vi "init Tests.vi"(8 "error in (no error)":errorcluster caption="Fehler (Eingang, kein Fehler)", 11 "EMTestCWS500N Eingang":refnum<class "EMTestCWS500N.lvclass"> caption="DNL_LabVIEW Object in") -> (0 "error out":errorcluster caption="Fehler (Ausgang)", 3 "EMTestCWS500N Ausgang":refnum<class "EMTestCWS500N.lvclass"> caption="DNL_LabVIEW Object out")   [LabVIEW 2013, in "EMTestCWS500N.lvclass"]
uses:
  EMTestCWS500N.lvclass
  Tests/HF-Felder/HF-Felder.lvclass
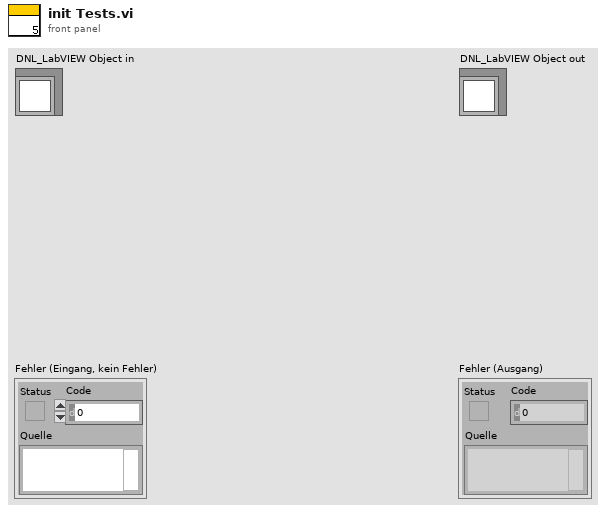
[diagram p1: front panel]
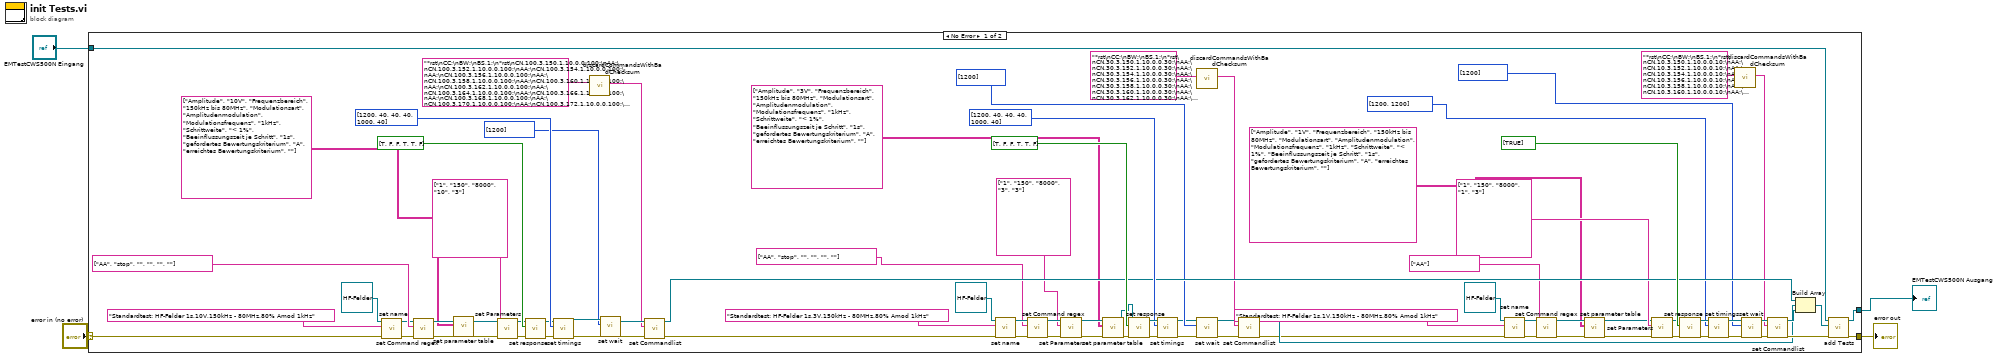
[diagram p0: block diagram]
diagram:
  n1 = case shown="No Error" "error in (no error)" {
    selector: "error in (no error)" -> [w52 w88]
    tunnel: [w76 w88] -> w4
    tunnel: "EMTestCWS500N Eingang" -> [w75 w89]
    tunnel: [w74 w89] -> w1
    frame No Error {
      n2 = call-dynamic "set name.vi"("error in (no error)"=w52, "name"="Standardtest: HF-Felder 1s,10V,150kHz - 80MHz,80% Amod 1kHz", "TestInterface (Eingang)"=refnum<class "HF-Felder.lvclass"> refnum ("HF-Felder.lvclass")) -> ("error out"=w51:errorcluster, "TestInterface (Ausgang)"=w57:refnum<class "HF-Felder.lvclass">)  [unwired: 7 in]
      n3 = call-dynamic "set Command regex.vi"("error in (no error)"=w51, "Command regex"=string[] ["AA", "stop", "", "", "", ""], "TestInterface (Eingang)"=w57) -> ("error out"=w30:errorcluster, "TestInterface (Ausgang)"=w31:refnum<class "HF-Felder.lvclass">)  [unwired: 7 in]
      n4 = call-dynamic "set parameter table.vi"("error in (no error)"=w30, "parameter table"=string[][] [["Amplitude", "10V"], ["Frequenzbereich", "150kHz bis 80MHz"], ["Modulationsart", "Amplitudenmodulation"], ["Modulationsfrequenz", "1kHz"], ["Schrittweite", "< 1%"], ["Beeinflussungszeit je Schritt", "1s"], ["gefordertes Bewertungskriterium", "A"], ["erreichtes Bewertungskriterium", ""]] ("parameters"), "TestInterface in"=w31) -> ("error out"=w29:errorcluster, "TestInterface out"=w28:refnum<class "HF-Felder.lvclass">)  [unwired: 7 in]
      n5 = call-dynamic "set Parameters.vi"("error in (no error)"=w29, "parameters"=string[] ["1", "150", "8000", "10", "3"], "TestInterface (Eingang)"=w28) -> ("error out"=w50:errorcluster, "TestInterface (Ausgang)"=w58:refnum<class "HF-Felder.lvclass">)  [unwired: 7 in]
      n6 = call-dynamic "set response.vi"("error in (no error)"=w50, "response?"=bool[] [TRUE, FALSE, FALSE, TRUE, TRUE, FALSE], "TestInterface (Eingang)"=w58) -> ("error out"=w49:errorcluster, "TestInterface (Ausgang)"=w59:refnum<class "HF-Felder.lvclass">)  [unwired: 7 in]
      n7 = call-dynamic "set timings.vi"("error in (no error)"=w49, "timings"=i32[] [1200, 40, 40, 40, 1000, 40] ("Timings"), "TestInterface (Eingang)"=w59) -> ("error out"=w40:errorcluster, "TestInterface (Ausgang)"=w37:refnum<class "HF-Felder.lvclass">)  [unwired: 7 in]
      n8 = call "discardCommandsWithBadChecksum.vi"("multi-line string"="*rst\nCC;\nBW;\nBS,1;\n*rst\nCN,100,3,150,1,10,0,0,100;\nAA;\nCN,100,3,152,1,10,0,0,100;\nAA;\nCN,100,3,154,1,10,0,0,100;\nAA;\nCN,100,3,156,1,10,0,0,100;\nAA;\nCN,100,3,158,1,10,0,0,100;\nAA;\nCN,100,3,160,1,10,0,0,100;\nAA;\nCN,100,3,162,1,10,0,0,100;\nAA;\nCN,100,3,164,1,10,0,0,100;\nAA;\nCN,100,3,166,1,10,0,0,100;\nAA;\nCN,100,3,168,1,10,0,0,100;\nAA;\nCN,100,3,170,1,10,0,0,100;\nAA;\nCN,100,3,172,1,10,0,0,100;\nAA;\nCN,100,3,174,1,10,0,0,100;\nAA;\nCN,100,3,176,1,10,0,0,100;\nAA;\nCN,100,3,178,1,10,0,0,100;\nAA;\nCN,100,3,180,1,10,0,0,100;\nAA;\nCN,100,3,182,1,10,0,0,100;\nAA;\nCN,100,3,184,1,10,0,0,100;\nAA;\nCN,100,3,186,1,10,0,0,100;\nAA;\nCN,100,3,188,1,10,0,0,100;\nAA;\nCN,100,3,190,1,10,0,0,100;\nAA;\nCN,100,3,192,1,10,0,0,100;\nAA;\nCN,100,3,194,1,10,0,0,100;\nAA;\nCN,100,3,196,1,10,0,0,100;\nAA;\nCN,100,3,198,1,10,0,0,100;\nAA;\nCN,100,3,200,1,10,0,0,100;\nAA;\nCN,100,3,202,1,10,0,0,100;\nAA;\nCN,100,3,204,1,10,0,0,100;\nAA;\nCN,100,3,206,1,10,0,0,100;\nAA;\nCN,100,3,208,1,10,0,0,100;\nAA;\nCN,100,3,210,1,10,0,0,100;\nAA;\nCN,100,3,212,1,10,0,0,100;\nAA;\nCN,100,3,214,1,10,0,0,100;\nAA;\nCN,100,3,216,1,10,0,0,100;\nAA;\nCN,100,3,218,1,10,0,0,100;\nAA;\nCN,100,3,220,1,10,0,0,100;\nAA;\nCN,100,3,222,1,10,0,0,100;\nAA;\nCN,100,3,224,1,10,0,0,100;\nAA;\nCN,100,3,226,1,10,0,0,100;\nAA;\nCN,100,3,228,1,10,0,0,100;\nAA;\nCN,100,3,230,1,10,0,0,100;\nAA;\nCN,100,3,232,1,10,0,0,100;\nAA;\nCN,100,3,234,1,10,0,0,100;\nAA;\nCN,100,3,236,1,10,0,0,100;\nAA;\nCN,100,3,238,1,10,0,0,100;\nAA;\nCN,100,3,240,1,10,0,0,100;\nAA;\nCN,100,3,242,1,10,0,0,100;\nAA;\nCN,100,3,244,1,10,0,0,100;\nAA;\nCN,100,3,246,1,10,0,0,100;\nAA;\nCN,100,3,248,1,10,0,0,100;\nAA;\nCN,100,3,250,1,10,0,0,100;\nAA;\nCN,100,3,252,1,10,0,0,100;\nAA;\nCN,100,3,255,1,10,0,0,100;\nAA;\nCN,100,3,258,1,10,0,0,100;\nAA;\nCN,100,3,261,1,10,0,0,100;\nAA;\nCN,100,3,264,1,10,0,0,100;\nAA;\nCN,100,3,267,1,10,0,0,100;\nAA;\nCN,100,3,270,1,10,0,0,100;\nAA;\nCN,100,3,273,1,10,0,0,100;\nAA;\nCN,100,3,276,1,10,0,0,100;\nAA;\nCN,100,3,279,1,10,0,0,100;\nAA;\nCN,100,3,282,1,10,0,0,100;\nAA;\nCN,100,3,285,1,10,0,0,100;\nAA;\nCN,100,3,288,1,10,0,0,100;\nAA;\nCN,100,3,291,1,10,0,0,100;\nAA;\nCN,100,3,294,1,10,0,0,100;\nAA;\nCN,100,3,297,1,10,0,0,100;\nAA;\nCN,100,3,300,1,10,0,0,100;\nAA;\nCN,100,3,303,1,10,0,0,100;\nAA;\nCN,100,3,306,1,10,0,0,100;\nAA;\nCN,100,3,309,1,10,0,0,100;\nAA;\nCN,100,3,312,1,10,0,0,100;\nAA;\nCN,100,3,315,1,10,0,0,100;\nAA;\nCN,100,3,318,1,10,0,0,100;\nAA;\nCN,100,3,321,1,10,0,0,100;\nAA;\nCN,100,3,324,1,10,0,0,100;\nAA;\nCN,100,3,327,1,10,0,0,100;\nAA;\nCN,100,3,330,1,10,0,0,100;\nAA;\nCN,100,3,333,1,10,0,0,100;\nAA;\nCN,100,3,336,1,10,0,0,100;\nAA;\nCN,100,3,339,1,10,0,0,100;\nAA;\nCN,100,3,342,1,10,0,0,100;\nAA;\nCN,100,3,345,1,10,0,0,100;\nAA;\nCN,100,3,348,1,10,0,0,100;\nAA;\nCN,100,3,351,1,10,0,0,100;\nAA;\nCN,100,3,355,1,10,0,0,100;\nAA;\nCN,100,3,359,1,10,0,0,100;\nAA;\nCN,100,3,363,1,10,0,0,100;\nAA;\nCN,100,3,367,1,10,0,0,100;\nAA;\nCN,100,3,371,1,10,0,0,100;\nAA;\nCN,100,3,375,1,10,0,0,100;\nAA;\nCN,100,3,379,1,10,0,0,100;\nAA;\nCN,100,3,383,1,10,0,0,100;\nAA;\nCN,100,3,387,1,10,0,0,100;\nAA;\nCN,100,3,391,1,10,0,0,100;\nAA;\nCN,100,3,395,1,10,0,0,100;\nAA;\nCN,100,3,399,1,10,0,0,100;\nAA;\nCN,100,3,403,1,10,0,0,100;\nAA;\nCN,100,3,407,1,10,0,0,100;\nAA;\nCN,100,3,411,1,10,0,0,100;\nAA;\nCN,100,3,415,1,10,0,0,100;\nAA;\nCN,100,3,419,1,10,0,0,100;\nAA;\nCN,100,3,423,1,10,0,0,100;\nAA;\nCN,100,3,427,1,10,0,0,100;\nAA;\nCN,100,3,431,1,10,0,0,100;\nAA;\nCN,100,3,435,1,10,0,0,100;\nAA;\nCN,100,3,439,1,10,0,0,100;\nAA;\nCN,100,3,443,1,10,0,0,100;\nAA;\nCN,100,3,447,1,10,0,0,100;\nAA;\nCN,100,3,451,1,10,0,0,100;\nAA;\nCN,100,3,456,1,10,0,0,100;\nAA;\nCN,100,3,461,1,10,0,0,100;\nAA;\nCN,100,3,466,1,10,0,0,100;\nAA;\nCN,100,3,471,1,10,0,0,100;\nAA;\nCN,100,3,476,1,10,0,0,100;\nAA;\nCN,100,3,481,1,10,0,0,100;\nAA;\nCN,100,3,486,1,10,0,0,100;\nAA;\nCN,100,3,491,1,10,0,0,100;\nAA;\nCN,100,3,496,1,10,0,0,100;\nAA;\nCN,100,3,501,1,10,0,0,100;\nAA;\nCN,100,3,506,1,10,0,0,100;\nAA;\nCN,100,3,511,1,10,0,0,100;\nAA;\nCN,100,3,516,1,10,0,0,100;\nAA;\nCN,100,3,521,1,10,0,0,100;\nAA;\nCN,100,3,526,1,10,0,0,100;\nAA;\nCN,100,3,531,1,10,0,0,100;\nAA;\nCN,100,3,536,1,10,0,0,100;\nAA;\nCN,100,3,541,1,10,0,0,100;\nAA;\nCN,100,3,546,1,10,0,0,100;\nAA;\nCN,100,3,551,1,10,0,0,100;\nAA;\nCN,100,3,557,1,10,0,0,100;\nAA;\nCN,100,3,563,1,10,0,0,100;\nAA;\nCN,100,3,569,1,10,0,0,100;\nAA;\nCN,100,3,575,1,10,0,0,100;\nAA;\nCN,100,3,581,1,10,0,0,100;\nAA;\nCN,100,3,587,1,10,0,0,100;\nAA;\nCN,100,3,593,1,10,0,0,100;\nAA;\nCN,100,3,599,1,10,0,0,100;\nAA;\nCN,100,3,605,1,10,0,0,100;\nAA;\nCN,100,3,611,1,10,0,0,100;\nAA;\nCN,100,3,617,1,10,0,0,100;\nAA;\nCN,100,3,623,1,10,0,0,100;\nAA;\nCN,100,3,629,1,10,0,0,100;\nAA;\nCN,100,3,635,1,10,0,0,100;\nAA;\nCN,100,3,641,1,10,0,0,100;\nAA;\nCN,100,3,647,1,10,0,0,100;\nAA;\nCN,100,3,653,1,10,0,0,100;\nAA;\nCN,100,3,660,1,10,0,0,100;\nAA;\nCN,100,3,667,1,10,0,0,100;\nAA;\nCN,100,3,674,1,10,0,0,100;\nAA;\nCN,100,3,681,1,10,0,0,100;\nAA;\nCN,100,3,688,1,10,0,0,100;\nAA;\nCN,100,3,695,1,10,0,0,100;\nAA;\nCN,100,3,702,1,10,0,0,100;\nAA;\nCN,100,3,709,1,10,0,0,100;\nAA;\nCN,100,3,716,1,10,0,0,100;\nAA;\nCN,100,3,723,1,10,0,0,100;\nAA;\nCN,100,3,730,1,10,0,0,100;\nAA;\nCN,100,3,737,1,10,0,0,100;\nAA;\nCN,100,3,744,1,10,0,0,100;\nAA;\nCN,100,3,751,1,10,0,0,100;\nAA;\nCN,100,3,759,1,10,0,0,100;\nAA;\nCN,100,3,767,1,10,0,0,100;\nAA;\nCN,100,3,775,1,10,0,0,100;\nAA;\nCN,100,3,783,1,10,0,0,100;\nAA;\nCN,100,3,791,1,10,0,0,100;\nAA;\nCN,100,3,799,1,10,0,0,100;\nAA;\nCN,100,3,807,1,10,0,0,100;\nAA;\nCN,100,3,815,1,10,0,0,100;\nAA;\nCN,100,3,823,1,10,0,0,100;\nAA;\nCN,100,3,831,1,10,0,0,100;\nAA;\nCN,100,3,839,1,10,0,0,100;\nAA;\nCN,100,3,847,1,10,0,0,100;\nAA;\nCN,100,3,855,1,10,0,0,100;\nAA;\nCN,100,3,864,1,10,0,0,100;\nAA;\nCN,100,3,873,1,10,0,0,100;\nAA;\nCN,100,3,882,1,10,0,0,100;\nAA;\nCN,100,3,891,1,10,0,0,100;\nAA;\nCN,100,3,900,1,10,0,0,100;\nAA;\nCN,100,3,909,1,10,0,0,100;\nAA;\nCN,100,3,918,1,10,0,0,100;\nAA;\nCN,100,3,927,1,10,0,0,100;\nAA;\nCN,100,3,936,1,10,0,0,100;\nAA;\nCN,100,3,945,1,10,0,0,100;\nAA;\nCN,100,3,954,1,10,0,0,100;\nAA;\nCN,100,3,964,1,10,0,0,100;\nAA;\nCN,100,3,974,1,10,0,0,100;\nAA;\nCN,100,3,984,1,10,0,0,100;\nAA;\nCN,100,3,994,1,10,0,0,100;\nAA;\nCN,100,3,1004,1,10,0,0,100;\nAA;\nCN,100,3,1014,1,10,0,0,100;\nAA;\nCN,100,3,1024,1,10,0,0,100;\nAA;\nCN,100,3,1034,1,10,0,0,100;\nAA;\nCN,100,3,1044,1,10,0,0,100;\nAA;\nCN,100,3,1054,1,10,0,0,100;\nAA;\nCN,100,3,1065,1,10,0,0,100;\nAA;\nCN,100,3,1076,1,10,0,0,100;\nAA;\nCN,100,3,1087,1,10,0,0,100;\nAA;\nCN,100,3,1098,1,10,0,0,100;\nAA;\nCN,100,3,1109,1,10,0,0,100;\nAA;\nCN,100,3,1120,1,10,0,0,100;\nAA;\nCN,100,3,1131,1,10,0,0,100;\nAA;\nCN,100,3,1142,1,10,0,0,100;\nAA;\nCN,100,3,1153,1,10,0,0,100;\nAA;\nCN,100,3,1165,1,10,0,0,100;\nAA;\nCN,100,3,1177,1,10,0,0,100;\nAA;\nCN,100,3,1189,1,10,0,0,100;\nAA;\nCN,100,3,1201,1,10,0,0,100;\nAA;\nCN,100,3,1213,1,10,0,0,100;\nAA;\nCN,100,3,1225,1,10,0,0,100;\nAA;\nCN,100,3,1237,1,10,0,0,100;\nAA;\nCN,100,3,1249,1,10,0,0,100;\nAA;\nCN,100,3,1261,1,10,0,0,100;\nAA;\nCN,100,3,1274,1,10,0,0,100;\nAA;\nCN,100,3,1287,1,10,0,0,100;\nAA;\nCN,100,3,1300,1,10,0,0,100;\nAA;\nCN,100,3,1313,1,10,0,0,100;\nAA;\nCN,100,3,1326,1,10,0,0,100;\nAA;\nCN,100,3,1339,1,10,0,0,100;\nAA;\nCN,100,3,1352,1,10,0,0,100;\nAA;\nCN,100,3,1366,1,10,0,0,100;\nAA;\nCN,100,3,1380,1,10,0,0,100;\nAA;\nCN,100,3,1394,1,10,0,0,100;\nAA;\nCN,100,3,1408,1,10,0,0,100;\nAA;\nCN,100,3,1422,1,10,0,0,100;\nAA;\nCN,100,3,1436,1,10,0,0,100;\nAA;\nCN,100,3,1450,1,10,0,0,100;\nAA;\nCN,100,3,1464,1,10,0,0,100;\nAA;\nCN,100,3,1479,1,10,0,0,100;\nAA;\nCN,100,3,1494,1,10,0,0,100;\nAA;\nCN,100,3,1509,1,10,0,0,100;\nAA;\nCN,100,3,1524,1,10,0,0,100;\nAA;\nCN,100,3,1539,1,10,0,0,100;\nAA;\nCN,100,3,1554,1,10,0,0,100;\nAA;\nCN,100,3,1570,1,10,0,0,100;\nAA;\nCN,100,3,1586,1,10,0,0,100;\nAA;\nCN,100,3,1602,1,10,0,0,100;\nAA;\nCN,100,3,1618,1,10,0,0,100;\nAA;\nCN,100,3,1634,1,10,0,0,100;\nAA;\nCN,100,3,1650,1,10,0,0,100;\nAA;\nCN,100,3,1666,1,10,0,0,100;\nAA;\nCN,100,3,1683,1,10,0,0,100;\nAA;\nCN,100,3,1700,1,10,0,0,100;\nAA;\nCN,100,3,1717,1,10,0,0,100;\nAA;\nCN,100,3,1734,1,10,0,0,100;\nAA;\nCN,100,3,1751,1,10,0,0,100;\nAA;\nCN,100,3,1769,1,10,0,0,100;\nAA;\nCN,100,3,1787,1,10,0,0,100;\nAA;\nCN,100,3,1805,1,10,0,0,100;\nAA;\nCN,100,3,1823,1,10,0,0,100;\nAA;\nCN,100,3,1841,1,10,0,0,100;\nAA;\nCN,100,3,1859,1,10,0,0,100;\nAA;\nCN,100,3,1878,1,10,0,0,100;\nAA;\nCN,100,3,1897,1,10,0,0,100;\nAA;\nCN,100,3,1916,1,10,0,0,100;\nAA;\nCN,100,3,1935,1,10,0,0,100;\nAA;\nCN,100,3,1954,1,10,0,0,100;\nAA;\nCN,100,3,1974,1,10,0,0,100;\nAA;\nCN,100,3,1994,1,10,0,0,100;\nAA;\nCN,100,3,2014,1,10,0,0,100;\nAA;\nCN,100,3,2034,1,10,0,0,100;\nAA;\nCN,100,3,2054,1,10,0,0,100;\nAA;\nCN,100,3,2075,1,10,0,0,100;\nAA;\nCN,100,3,2096,1,10,0,0,100;\nAA;\nCN,100,3,2117,1,10,0,0,100;\nAA;\nCN,100,3,2138,1,10,0,0,100;\nAA;\nCN,100,3,2159,1,10,0,0,100;\nAA;\nCN,100,3,2181,1,10,0,0,100;\nAA;\nCN,100,3,2203,1,10,0,0,100;\nAA;\nCN,100,3,2225,1,10,0,0,100;\nAA;\nCN,100,3,2247,1,10,0,0,100;\nAA;\nCN,100,3,2269,1,10,0,0,100;\nAA;\nCN,100,3,2292,1,10,0,0,100;\nAA;\nCN,100,3,2315,1,10,0,0,100;\nAA;\nCN,100,3,2338,1,10,0,0,100;\nAA;\nCN,100,3,2361,1,10,0,0,100;\nAA;\nCN,100,3,2385,1,10,0,0,100;\nAA;\nCN,100,3,2409,1,10,0,0,100;\nAA;\nCN,100,3,2433,1,10,0,0,100;\nAA;\nCN,100,3,2457,1,10,0,0,100;\nAA;\nCN,100,3,2482,1,10,0,0,100;\nAA;\nCN,100,3,2507,1,10,0,0,100;\nAA;\nCN,100,3,2532,1,10,0,0,100;\nAA;\nCN,100,3,2557,1,10,0,0,100;\nAA;\nCN,100,3,2583,1,10,0,0,100;\nAA;\nCN,100,3,2609,1,10,0,0,100;\nAA;\nCN,100,3,2635,1,10,0,0,100;\nAA;\nCN,100,3,2661,1,10,0,0,100;\nAA;\nCN,100,3,2688,1,10,0,0,100;\nAA;\nCN,100,3,2715,1,10,0,0,100;\nAA;\nCN,100,3,2742,1,10,0,0,100;\nAA;\nCN,100,3,2769,1,10,0,0,100;\nAA;\nCN,100,3,2797,1,10,0,0,100;\nAA;\nCN,100,3,2825,1,10,0,0,100;\nAA;\nCN,100,3,2853,1,10,0,0,100;\nAA;\nCN,100,3,2882,1,10,0,0,100;\nAA;\nCN,100,3,2911,1,10,0,0,100;\nAA;\nCN,100,3,2940,1,10,0,0,100;\nAA;\nCN,100,3,2969,1,10,0,0,100;\nAA;\nCN,100,3,2999,1,10,0,0,100;\nAA;\nCN,100,3,3029,1,10,0,0,100;\nAA;\nCN,100,3,3059,1,10,0,0,100;\nAA;\nCN,100,3,3090,1,10,0,0,100;\nAA;\nCN,100,3,3121,1,10,0,0,100;\nAA;\nCN,100,3,3152,1,10,0,0,100;\nAA;\nCN,100,3,3184,1,10,0,0,100;\nAA;\nCN,100,3,3216,1,10,0,0,100;\nAA;\nCN,100,3,3248,1,10,0,0,100;\nAA;\nCN,100,3,3280,1,10,0,0,100;\nAA;\nCN,100,3,3313,1,10,0,0,100;\nAA;\nCN,100,3,3346,1,10,0,0,100;\nAA;\nCN,100,3,3379,1,10,0,0,100;\nAA;\nCN,100,3,3413,1,10,0,0,100;\nAA;\nCN,100,3,3447,1,10,0,0,100;\nAA;\nCN,100,3,3481,1,10,0,0,100;\nAA;\nCN,100,3,3516,1,10,0,0,100;\nAA;\nCN,100,3,3551,1,10,0,0,100;\nAA;\nCN,100,3,3587,1,10,0,0,100;\nAA;\nCN,100,3,3623,1,10,0,0,100;\nAA;\nCN,100,3,3659,1,10,0,0,100;\nAA;\nCN,100,3,3696,1,10,0,0,100;\nAA;\nCN,100,3,3733,1,10,0,0,100;\nAA;\nCN,100,3,3770,1,10,0,0,100;\nAA;\nCN,100,3,3808,1,10,0,0,100;\nAA;\nCN,100,3,3846,1,10,0,0,100;\nAA;\nCN,100,3,3884,1,10,0,0,100;\nAA;\nCN,100,3,3923,1,10,0,0,100;\nAA;\nCN,100,3,3962,1,10,0,0,100;\nAA;\nCN,100,3,4002,1,10,0,0,100;\nAA;\nCN,100,3,4042,1,10,0,0,100;\nAA;\nCN,100,3,4082,1,10,0,0,100;\nAA;\nCN,100,3,4123,1,10,0,0,100;\nAA;\nCN,100,3,4164,1,10,0,0,100;\nAA;\nCN,100,3,4206,1,10,0,0,100;\nAA;\nCN,100,3,4248,1,10,0,0,100;\nAA;\nCN,100,3,4290,1,10,0,0,100;\nAA;\nCN,100,3,4333,1,10,0,0,100;\nAA;\nCN,100,3,4376,1,10,0,0,100;\nAA;\nCN,100,3,4420,1,10,0,0,100;\nAA;\nCN,100,3,4464,1,10,0,0,100;\nAA;\nCN,100,3,4509,1,10,0,0,100;\nAA;\nCN,100,3,4554,1,10,0,0,100;\nAA;\nCN,100,3,4600,1,10,0,0,100;\nAA;\nCN,100,3,4646,1,10,0,0,100;\nAA;\nCN,100,3,4692,1,10,0,0,100;\nAA;\nCN,100,3,4739,1,10,0,0,100;\nAA;\nCN,100,3,4786,1,10,0,0,100;\nAA;\nCN,100,3,4834,1,10,0,0,100;\nAA;\nCN,100,3,4882,1,10,0,0,100;\nAA;\nCN,100,3,4931,1,10,0,0,100;\nAA;\nCN,100,3,4980,1,10,0,0,100;\nAA;\nCN,100,3,5030,1,10,0,0,100;\nAA;\nCN,100,3,5080,1,10,0,0,100;\nAA;\nCN,100,3,5131,1,10,0,0,100;\nAA;\nCN,100,3,5182,1,10,0,0,100;\nAA;\nCN,100,3,5234,1,10,0,0,100;\nAA;\nCN,100,3,5286,1,10,0,0,100;\nAA;\nCN,100,3,5339,1,10,0,0,100;\nAA;\nCN,100,3,5392,1,10,0,0,100;\nAA;\nCN,100,3,5446,1,10,0,0,100;\nAA;\nCN,100,3,5500,1,10,0,0,100;\nAA;\nCN,100,3,5555,1,10,0,0,100;\nAA;\nCN,100,3,5611,1,10,0,0,100;\nAA;\nCN,100,3,5667,1,10,0,0,100;\nAA;\nCN,100,3,5724,1,10,0,0,100;\nAA;\nCN,100,3,5781,1,10,0,0,100;\nAA;\nCN,100,3,5839,1,10,0,0,100;\nAA;\nCN,100,3,5897,1,10,0,0,100;\nAA;\nCN,100,3,5956,1,10,0,0,100;\nAA;\nCN,100,3,6016,1,10,0,0,100;\nAA;\nCN,100,3,6076,1,10,0,0,100;\nAA;\nCN,100,3,6137,1,10,0,0,100;\nAA;\nCN,100,3,6198,1,10,0,0,100;\nAA;\nCN,100,3,6260,1,10,0,0,100;\nAA;\nCN,100,3,6323,1,10,0,0,100;\nAA;\nCN,100,3,6386,1,10,0,0,100;\nAA;\nCN,100,3,6450,1,10,0,0,100;\nAA;\nCN,100,3,6514,1,10,0,0,100;\nAA;\nCN,100,3,6579,1,10,0,0,100;\nAA;\nCN,100,3,6645,1,10,0,0,100;\nAA;\nCN,100,3,6711,1,10,0,0,100;\nAA;\nCN,100,3,6778,1,10,0,0,100;\nAA;\nCN,100,3,6846,1,10,0,0,100;\nAA;\nCN,100,3,6914,1,10,0,0,100;\nAA;\nCN,100,3,6983,1,10,0,0,100;\nAA;\nCN,100,3,7053,1,10,0,0,100;\nAA;\nCN,100,3,7124,1,10,0,0,100;\nAA;\nCN,100,3,7195,1,10,0,0,100;\nAA;\nCN,100,3,7267,1,10,0,0,100;\nAA;\nCN,100,3,7340,1,10,0,0,100;\nAA;\nCN,100,3,7413,1,10,0,0,100;\nAA;\nCN,100,3,7487,1,10,0,0,100;\nAA;\nCN,100,3,7562,1,10,0,0,100;\nAA;\nCN,100,3,7638,1,10,0,0,100;\nAA;\nCN,100,3,7714,1,10,0,0,100;\nAA;\nCN,100,3,7791,1,10,0,0,100;\nAA;\nCN,100,3,7869,1,10,0,0,100;\nAA;\nCN,100,3,7948,1,10,0,0,100;\nAA;\nCN,100,3,8027,1,10,0,0,100;\nAA;\nCN,100,3,8107,1,10,0,0,100;\nAA;\nCN,100,3,8188,1,10,0,0,100;\nAA;\nCN,100,3,8270,1,10,0,0,100;\nAA;\nCN,100,3,8353,1,10,0,0,100;\nAA;\nCN,100,3,8437,1,10,0,0,100;\nAA;\nCN,100,3,8521,1,10,0,0,100;\nAA;\nCN,100,3,8606,1,10,0,0,100;\nAA;\nCN,100,3,8692,1,10,0,0,100;\nAA;\nCN,100,3,8779,1,10,0,0,100;\nAA;\nCN,100,3,8867,1,10,0,0,100;\nAA;\nCN,100,3,8956,1,10,0,0,100;\nAA;\nCN,100,3,9046,1,10,0,0,100;\nAA;\nCN,100,3,9136,1,10,0,0,100;\nAA;\nCN,100,3,9227,1,10,0,0,100;\nAA;\nCN,100,3,9319,1,10,0,0,100;\nAA;\nCN,100,3,9412,1,10,0,0,100;\nAA;\nCN,100,3,9506,1,10,0,0,100;\nAA;\nCN,100,3,9601,1,10,0,0,100;\nAA;\nCN,100,3,9697,1,10,0,0,100;\nAA;\nCN,100,3,9794,1,10,0,0,100;\nAA;\nCN,100,3,9892,1,10,0,0,100;\nAA;\nCN,100,3,9991,1,10,0,0,100;\nAA;\nCN,100,3,10091,1,10,0,0,100;\nAA;\nCN,100,3,10192,1,10,0,0,100;\nAA;\nCN,100,3,10294,1,10,0,0,100;\nAA;\nCN,100,3,10397,1,10,0,0,100;\nAA;\nCN,100,3,10501,1,10,0,0,100;\nAA;\nCN,100,3,10606,1,10,0,0,100;\nAA;\nCN,100,3,10712,1,10,0,0,100;\nAA;\nCN,100,3,10819,1,10,0,0,100;\nAA;\nCN,100,3,10927,1,10,0,0,100;\nAA;\nCN,100,3,11036,1,10,0,0,100;\nAA;\nCN,100,3,11146,1,10,0,0,100;\nAA;\nCN,100,3,11257,1,10,0,0,100;\nAA;\nCN,100,3,11370,1,10,0,0,100;\nAA;\nCN,100,3,11484,1,10,0,0,100;\nAA;\nCN,100,3,11599,1,10,0,0,100;\nAA;\nCN,100,3,11715,1,10,0,0,100;\nAA;\nCN,100,3,11832,1,10,0,0,100;\nAA;\nCN,100,3,11950,1,10,0,0,100;\nAA;\nCN,100,3,12070,1,10,0,0,100;\nAA;\nCN,100,3,12191,1,10,0,0,100;\nAA;\nCN,100,3,12313,1,10,0,0,100;\nAA;\nCN,100,3,12436,1,10,0,0,100;\nAA;\nCN,100,3,12560,1,10,0,0,100;\nAA;\nCN,100,3,12686,1,10,0,0,100;\nAA;\nCN,100,3,12813,1,10,0,0,100;\nAA;\nCN,100,3,12941,1,10,0,0,100;\nAA;\nCN,100,3,13070,1,10,0,0,100;\nAA;\nCN,100,3,13201,1,10,0,0,100;\nAA;\nCN,100,3,13333,1,10,0,0,100;\nAA;\nCN,100,3,13466,1,10,0,0,100;\nAA;\nCN,100,3,13601,1,10,0,0,100;\nAA;\nCN,100,3,13737,1,10,0,0,100;\nAA;\nCN,100,3,13874,1,10,0,0,100;\nAA;\nCN,100,3,14013,1,10,0,0,100;\nAA;\nCN,100,3,14153,1,10,0,0,100;\nAA;\nCN,100,3,14295,1,10,0,0,100;\nAA;\nCN,100,3,14438,1,10,0,0,100;\nAA;\nCN,100,3,14582,1,10,0,0,100;\nAA;\nCN,100,3,14728,1,10,0,0,100;\nAA;\nCN,100,3,14875,1,10,0,0,100;\nAA;\nCN,100,3,15024,1,10,0,0,100;\nAA;\nCN,100,3,15174,1,10,0,0,100;\nAA;\nCN,100,3,15326,1,10,0,0,100;\nAA;\nCN,100,3,15479,1,10,0,0,100;\nAA;\nCN,100,3,15634,1,10,0,0,100;\nAA;\nCN,100,3,15790,1,10,0,0,100;\nAA;\nCN,100,3,15948,1,10,0,0,100;\nAA;\nCN,100,3,16107,1,10,0,0,100;\nAA;\nCN,100,3,16268,1,10,0,0,100;\nAA;\nCN,100,3,16431,1,10,0,0,100;\nAA;\nCN,100,3,16595,1,10,0,0,100;\nAA;\nCN,100,3,16761,1,10,0,0,100;\nAA;\nCN,100,3,16929,1,10,0,0,100;\nAA;\nCN,100,3,17098,1,10,0,0,100;\nAA;\nCN,100,3,17269,1,10,0,0,100;\nAA;\nCN,100,3,17442,1,10,0,0,100;\nAA;\nCN,100,3,17616,1,10,0,0,100;\nAA;\nCN,100,3,17792,1,10,0,0,100;\nAA;\nCN,100,3,17970,1,10,0,0,100;\nAA;\nCN,100,3,18150,1,10,0,0,100;\nAA;\nCN,100,3,18332,1,10,0,0,100;\nAA;\nCN,100,3,18515,1,10,0,0,100;\nAA;\nCN,100,3,18700,1,10,0,0,100;\nAA;\nCN,100,3,18887,1,10,0,0,100;\nAA;\nCN,100,3,19076,1,10,0,0,100;\nAA;\nCN,100,3,19267,1,10,0,0,100;\nAA;\nCN,100,3,19460,1,10,0,0,100;\nAA;\nCN,100,3,19655,1,10,0,0,100;\nAA;\nCN,100,3,19852,1,10,0,0,100;\nAA;\nCN,100,3,20051,1,10,0,0,100;\nAA;\nCN,100,3,20252,1,10,0,0,100;\nAA;\nCN,100,3,20455,1,10,0,0,100;\nAA;\nCN,100,3,20660,1,10,0,0,100;\nAA;\nCN,100,3,20867,1,10,0,0,100;\nAA;\nCN,100,3,21076,1,10,0,0,100;\nAA;\nCN,100,3,21287,1,10,0,0,100;\nAA;\nCN,100,3,21500,1,10,0,0,100;\nAA;\nCN,100,3,21715,1,10,0,0,100;\nAA;\nCN,100,3,21932,1,10,0,0,100;\nAA;\nCN,100,3,22151,1,10,0,0,100;\nAA;\nCN,100,3,22373,1,10,0,0,100;\nAA;\nCN,100,3,22597,1,10,0,0,100;\nAA;\nCN,100,3,22823,1,10,0,0,100;\nAA;\nCN,100,3,23051,1,10,0,0,100;\nAA;\nCN,100,3,23282,1,10,0,0,100;\nAA;\nCN,100,3,23515,1,10,0,0,100;\nAA;\nCN,100,3,23750,1,10,0,0,100;\nAA;\nCN,100,3,23988,1,10,0,0,100;\nAA;\nCN,100,3,24228,1,10,0,0,100;\nAA;\nCN,100,3,24470,1,10,0,0,100;\nAA;\nCN,100,3,24715,1,10,0,0,100;\nAA;\nCN,100,3,24962,1,10,0,0,100;\nAA;\nCN,100,3,25212,1,10,0,0,100;\nAA;\nCN,100,3,25464,1,10,0,0,100;\nAA;\nCN,100,3,25719,1,10,0,0,100;\nAA;\nCN,100,3,25976,1,10,0,0,100;\nAA;\nCN,100,3,26236,1,10,0,0,100;\nAA;\nCN,100,3,26498,1,10,0,0,100;\nAA;\nCN,100,3,26763,1,10,0,0,100;\nAA;\nCN,100,3,27031,1,10,0,0,100;\nAA;\nCN,100,3,27301,1,10,0,0,100;\nAA;\nCN,100,3,27574,1,10,0,0,100;\nAA;\nCN,100,3,27850,1,10,0,0,100;\nAA;\nCN,100,3,28128,1,10,0,0,100;\nAA;\nCN,100,3,28409,1,10,0,0,100;\nAA;\nCN,100,3,28693,1,10,0,0,100;\nAA;\nCN,100,3,28980,1,10,0,0,100;\nAA;\nCN,100,3,29270,1,10,0,0,100;\nAA;\nCN,100,3,29563,1,10,0,0,100;\nAA;\nCN,100,3,29859,1,10,0,0,100;\nAA;\nCN,100,3,30158,1,10,0,0,100;\nAA;\nCN,100,3,30460,1,10,0,0,100;\nAA;\nCN,100,3,30765,1,10,0,0,100;\nAA;\nCN,100,3,31073,1,10,0,0,100;\nAA;\nCN,100,3,31384,1,10,0,0,100;\nAA;\nCN,100,3,31698,1,10,0,0,100;\nAA;\nCN,100,3,32015,1,10,0,0,100;\nAA;\nCN,100,3,32335,1,10,0,0,100;\nAA;\nCN,100,3,32658,1,10,0,0,100;\nAA;\nCN,100,3,32985,1,10,0,0,100;\nAA;\nCN,100,3,33315,1,10,0,0,100;\nAA;\nCN,100,3,33648,1,10,0,0,100;\nAA;\nCN,100,3,33984,1,10,0,0,100;\nAA;\nCN,100,3,34324,1,10,0,0,100;\nAA;\nCN,100,3,34667,1,10,0,0,100;\nAA;\nCN,100,3,35014,1,10,0,0,100;\nAA;\nCN,100,3,35364,1,10,0,0,100;\nAA;\nCN,100,3,35718,1,10,0,0,100;\nAA;\nCN,100,3,36075,1,10,0,0,100;\nAA;\nCN,100,3,36436,1,10,0,0,100;\nAA;\nCN,100,3,36800,1,10,0,0,100;\nAA;\nCN,100,3,37168,1,10,0,0,100;\nAA;\nCN,100,3,37540,1,10,0,0,100;\nAA;\nCN,100,3,37915,1,10,0,0,100;\nAA;\nCN,100,3,38294,1,10,0,0,100;\nAA;\nCN,100,3,38677,1,10,0,0,100;\nAA;\nCN,100,3,39064,1,10,0,0,100;\nAA;\nCN,100,3,39455,1,10,0,0,100;\nAA;\nCN,100,3,39850,1,10,0,0,100;\nAA;\nCN,100,3,40248,1,10,0,0,100;\nAA;\nCN,100,3,40650,1,10,0,0,100;\nAA;\nCN,100,3,41056,1,10,0,0,100;\nAA;\nCN,100,3,41467,1,10,0,0,100;\nAA;\nCN,100,3,41882,1,10,0,0,100;\nAA;\nCN,100,3,42301,1,10,0,0,100;\nAA;\nCN,100,3,42724,1,10,0,0,100;\nAA;\nCN,100,3,43151,1,10,0,0,100;\nAA;\nCN,100,3,43583,1,10,0,0,100;\nAA;\nCN,100,3,44019,1,10,0,0,100;\nAA;\nCN,100,3,44459,1,10,0,0,100;\nAA;\nCN,100,3,44904,1,10,0,0,100;\nAA;\nCN,100,3,45353,1,10,0,0,100;\nAA;\nCN,100,3,45807,1,10,0,0,100;\nAA;\nCN,100,3,46265,1,10,0,0,100;\nAA;\nCN,100,3,46728,1,10,0,0,100;\nAA;\nCN,100,3,47195,1,10,0,0,100;\nAA;\nCN,100,3,47667,1,10,0,0,100;\nAA;\nCN,100,3,48144,1,10,0,0,100;\nAA;\nCN,100,3,48625,1,10,0,0,100;\nAA;\nCN,100,3,49111,1,10,0,0,100;\nAA;\nCN,100,3,49602,1,10,0,0,100;\nAA;\nCN,100,3,50098,1,10,0,0,100;\nAA;\nCN,100,3,50599,1,10,0,0,100;\nAA;\nCN,100,3,51105,1,10,0,0,100;\nAA;\nCN,100,3,51616,1,10,0,0,100;\nAA;\nCN,100,3,52132,1,10,0,0,100;\nAA;\nCN,100,3,52653,1,10,0,0,100;\nAA;\nCN,100,3,53180,1,10,0,0,100;\nAA;\nCN,100,3,53712,1,10,0,0,100;\nAA;\nCN,100,3,54249,1,10,0,0,100;\nAA;\nCN,100,3,54791,1,10,0,0,100;\nAA;\nCN,100,3,55339,1,10,0,0,100;\nAA;\nCN,100,3,55892,1,10,0,0,100;\nAA;\nCN,100,3,56451,1,10,0,0,100;\nAA;\nCN,100,3,57016,1,10,0,0,100;\nAA;\nCN,100,3,57586,1,10,0,0,100;\nAA;\nCN,100,3,58162,1,10,0,0,100;\nAA;\nCN,100,3,58744,1,10,0,0,100;\nAA;\nCN,100,3,59331,1,10,0,0,100;\nAA;\nCN,100,3,59924,1,10,0,0,100;\nAA;\nCN,100,3,60523,1,10,0,0,100;\nAA;\nCN,100,3,61128,1,10,0,0,100;\nAA;\nCN,100,3,61739,1,10,0,0,100;\nAA;\nCN,100,3,62356,1,10,0,0,100;\nAA;\nCN,100,3,62980,1,10,0,0,100;\nAA;\nCN,100,3,63610,1,10,0,0,100;\nAA;\nCN,100,3,64246,1,10,0,0,100;\nAA;\nCN,100,3,64888,1,10,0,0,100;\nAA;\nCN,100,3,65537,1,10,0,0,100;\nAA;\nCN,100,3,66192,1,10,0,0,100;\nAA;\nCN,100,3,66854,1,10,0,0,100;\nAA;\nCN,100,3,67523,1,10,0,0,100;\nAA;\nCN,100,3,68198,1,10,0,0,100;\nAA;\nCN,100,3,68880,1,10,0,0,100;\nAA;\nCN,100,3,69569,1,10,0,0,100;\nAA;\nCN,100,3,70265,1,10,0,0,100;\nAA;\nCN,100,3,70968,1,10,0,0,100;\nAA;\nCN,100,3,71678,1,10,0,0,100;\nAA;\nCN,100,3,72395,1,10,0,0,100;\nAA;\nCN,100,3,73119,1,10,0,0,100;\nAA;\nCN,100,3,73850,1,10,0,0,100;\nAA;\nCN,100,3,74588,1,10,0,0,100;\nAA;\nCN,100,3,75334,1,10,0,0,100;\nAA;\nCN,100,3,76087,1,10,0,0,100;\nAA;\nCN,100,3,76848,1,10,0,0,100;\nAA;\nCN,100,3,77616,1,10,0,0,100;\nAA;\nCN,100,3,78392,1,10,0,0,100;\nAA;\nCN,100,3,79176,1,10,0,0,100;\nAA;\nCN,100,3,79968,1,10,0,0,100;\nAA;\nCN,100,3,80000,1,10,0,0,100;\nAA;\nAR;" ("Commandlist")) -> ("outputstring"=w10:string)  [unwired: 10 in]
      n9 = call-dynamic "set wait.vi"("error in (no error)"=w40, "wait"=i32[] [1200], "TestInterface in"=w37) -> ("error out"=w39:errorcluster, "TestInterface out"=w38:refnum<class "HF-Felder.lvclass">)  [unwired: 7 in]
      n10 = call-dynamic "set Commandlist.vi"("error in (no error)"=w39, "Commandlist"=w10, "TestInterface (Eingang)"=w38) -> ("error out"=w48:errorcluster, "TestInterface (Ausgang)"=w55:refnum<class "HF-Felder.lvclass">)  [unwired: 7 in]
      n11 = call-dynamic "set name.vi"("error in (no error)"=w48, "name"="Standardtest: HF-Felder 1s,3V,150kHz - 80MHz,80% Amod 1kHz", "TestInterface (Eingang)"=refnum<class "HF-Felder.lvclass"> refnum ("HF-Felder.lvclass")) -> ("error out"=w69:errorcluster, "TestInterface (Ausgang)"=w71:refnum<class "HF-Felder.lvclass">)  [unwired: 7 in]
      n12 = call-dynamic "set Command regex.vi"("error in (no error)"=w69, "Command regex"=string[] ["AA", "stop", "", "", "", ""], "TestInterface (Eingang)"=w71) -> ("error out"=w25:errorcluster, "TestInterface (Ausgang)"=w24:refnum<class "HF-Felder.lvclass">)  [unwired: 7 in]
      n13 = call-dynamic "set Parameters.vi"("error in (no error)"=w25, "parameters"=string[] ["1", "150", "8000", "3", "3"], "TestInterface (Eingang)"=w24) -> ("error out"=w18:errorcluster, "TestInterface (Ausgang)"=w20:refnum<class "HF-Felder.lvclass">)  [unwired: 7 in]
      n14 = call-dynamic "set parameter table.vi"("error in (no error)"=w18, "parameter table"=string[][] [["Amplitude", "3V"], ["Frequenzbereich", "150kHz bis 80MHz"], ["Modulationsart", "Amplitudenmodulation"], ["Modulationsfrequenz", "1kHz"], ["Schrittweite", "< 1%"], ["Beeinflussungszeit je Schritt", "1s"], ["gefordertes Bewertungskriterium", "A"], ["erreichtes Bewertungskriterium", ""]] ("parameters"), "TestInterface in"=w20) -> ("error out"=w22:errorcluster, "TestInterface out"=w21:refnum<class "HF-Felder.lvclass">)  [unwired: 7 in]
      n15 = call-dynamic "set response.vi"("error in (no error)"=w22, "response?"=bool[] [TRUE, FALSE, FALSE, TRUE, TRUE, FALSE], "TestInterface (Eingang)"=w21) -> ("error out"=w68:errorcluster, "TestInterface (Ausgang)"=w70:refnum<class "HF-Felder.lvclass">)  [unwired: 7 in]
      n16 = call-dynamic "set timings.vi"("error in (no error)"=w68, "timings"=i32[] [1200, 40, 40, 40, 1000, 40] ("Timings"), "TestInterface (Eingang)"=w70) -> ("error out"=w33:errorcluster, "TestInterface (Ausgang)"=w34:refnum<class "HF-Felder.lvclass">)  [unwired: 7 in]
      n17 = call "discardCommandsWithBadChecksum.vi"("multi-line string"="*rst\nCC;\nBW;\nBS,1;\n*rst\nCN,30,3,150,1,10,0,0,30;\nAA;\nCN,30,3,152,1,10,0,0,30;\nAA;\nCN,30,3,154,1,10,0,0,30;\nAA;\nCN,30,3,156,1,10,0,0,30;\nAA;\nCN,30,3,158,1,10,0,0,30;\nAA;\nCN,30,3,160,1,10,0,0,30;\nAA;\nCN,30,3,162,1,10,0,0,30;\nAA;\nCN,30,3,164,1,10,0,0,30;\nAA;\nCN,30,3,166,1,10,0,0,30;\nAA;\nCN,30,3,168,1,10,0,0,30;\nAA;\nCN,30,3,170,1,10,0,0,30;\nAA;\nCN,30,3,172,1,10,0,0,30;\nAA;\nCN,30,3,174,1,10,0,0,30;\nAA;\nCN,30,3,176,1,10,0,0,30;\nAA;\nCN,30,3,178,1,10,0,0,30;\nAA;\nCN,30,3,180,1,10,0,0,30;\nAA;\nCN,30,3,182,1,10,0,0,30;\nAA;\nCN,30,3,184,1,10,0,0,30;\nAA;\nCN,30,3,186,1,10,0,0,30;\nAA;\nCN,30,3,188,1,10,0,0,30;\nAA;\nCN,30,3,190,1,10,0,0,30;\nAA;\nCN,30,3,192,1,10,0,0,30;\nAA;\nCN,30,3,194,1,10,0,0,30;\nAA;\nCN,30,3,196,1,10,0,0,30;\nAA;\nCN,30,3,198,1,10,0,0,30;\nAA;\nCN,30,3,200,1,10,0,0,30;\nAA;\nCN,30,3,202,1,10,0,0,30;\nAA;\nCN,30,3,204,1,10,0,0,30;\nAA;\nCN,30,3,206,1,10,0,0,30;\nAA;\nCN,30,3,208,1,10,0,0,30;\nAA;\nCN,30,3,210,1,10,0,0,30;\nAA;\nCN,30,3,212,1,10,0,0,30;\nAA;\nCN,30,3,214,1,10,0,0,30;\nAA;\nCN,30,3,216,1,10,0,0,30;\nAA;\nCN,30,3,218,1,10,0,0,30;\nAA;\nCN,30,3,220,1,10,0,0,30;\nAA;\nCN,30,3,222,1,10,0,0,30;\nAA;\nCN,30,3,224,1,10,0,0,30;\nAA;\nCN,30,3,226,1,10,0,0,30;\nAA;\nCN,30,3,228,1,10,0,0,30;\nAA;\nCN,30,3,230,1,10,0,0,30;\nAA;\nCN,30,3,232,1,10,0,0,30;\nAA;\nCN,30,3,234,1,10,0,0,30;\nAA;\nCN,30,3,236,1,10,0,0,30;\nAA;\nCN,30,3,238,1,10,0,0,30;\nAA;\nCN,30,3,240,1,10,0,0,30;\nAA;\nCN,30,3,242,1,10,0,0,30;\nAA;\nCN,30,3,244,1,10,0,0,30;\nAA;\nCN,30,3,246,1,10,0,0,30;\nAA;\nCN,30,3,248,1,10,0,0,30;\nAA;\nCN,30,3,250,1,10,0,0,30;\nAA;\nCN,30,3,252,1,10,0,0,30;\nAA;\nCN,30,3,255,1,10,0,0,30;\nAA;\nCN,30,3,258,1,10,0,0,30;\nAA;\nCN,30,3,261,1,10,0,0,30;\nAA;\nCN,30,3,264,1,10,0,0,30;\nAA;\nCN,30,3,267,1,10,0,0,30;\nAA;\nCN,30,3,270,1,10,0,0,30;\nAA;\nCN,30,3,273,1,10,0,0,30;\nAA;\nCN,30,3,276,1,10,0,0,30;\nAA;\nCN,30,3,279,1,10,0,0,30;\nAA;\nCN,30,3,282,1,10,0,0,30;\nAA;\nCN,30,3,285,1,10,0,0,30;\nAA;\nCN,30,3,288,1,10,0,0,30;\nAA;\nCN,30,3,291,1,10,0,0,30;\nAA;\nCN,30,3,294,1,10,0,0,30;\nAA;\nCN,30,3,297,1,10,0,0,30;\nAA;\nCN,30,3,300,1,10,0,0,30;\nAA;\nCN,30,3,303,1,10,0,0,30;\nAA;\nCN,30,3,306,1,10,0,0,30;\nAA;\nCN,30,3,309,1,10,0,0,30;\nAA;\nCN,30,3,312,1,10,0,0,30;\nAA;\nCN,30,3,315,1,10,0,0,30;\nAA;\nCN,30,3,318,1,10,0,0,30;\nAA;\nCN,30,3,321,1,10,0,0,30;\nAA;\nCN,30,3,324,1,10,0,0,30;\nAA;\nCN,30,3,327,1,10,0,0,30;\nAA;\nCN,30,3,330,1,10,0,0,30;\nAA;\nCN,30,3,333,1,10,0,0,30;\nAA;\nCN,30,3,336,1,10,0,0,30;\nAA;\nCN,30,3,339,1,10,0,0,30;\nAA;\nCN,30,3,342,1,10,0,0,30;\nAA;\nCN,30,3,345,1,10,0,0,30;\nAA;\nCN,30,3,348,1,10,0,0,30;\nAA;\nCN,30,3,351,1,10,0,0,30;\nAA;\nCN,30,3,355,1,10,0,0,30;\nAA;\nCN,30,3,359,1,10,0,0,30;\nAA;\nCN,30,3,363,1,10,0,0,30;\nAA;\nCN,30,3,367,1,10,0,0,30;\nAA;\nCN,30,3,371,1,10,0,0,30;\nAA;\nCN,30,3,375,1,10,0,0,30;\nAA;\nCN,30,3,379,1,10,0,0,30;\nAA;\nCN,30,3,383,1,10,0,0,30;\nAA;\nCN,30,3,387,1,10,0,0,30;\nAA;\nCN,30,3,391,1,10,0,0,30;\nAA;\nCN,30,3,395,1,10,0,0,30;\nAA;\nCN,30,3,399,1,10,0,0,30;\nAA;\nCN,30,3,403,1,10,0,0,30;\nAA;\nCN,30,3,407,1,10,0,0,30;\nAA;\nCN,30,3,411,1,10,0,0,30;\nAA;\nCN,30,3,415,1,10,0,0,30;\nAA;\nCN,30,3,419,1,10,0,0,30;\nAA;\nCN,30,3,423,1,10,0,0,30;\nAA;\nCN,30,3,427,1,10,0,0,30;\nAA;\nCN,30,3,431,1,10,0,0,30;\nAA;\nCN,30,3,435,1,10,0,0,30;\nAA;\nCN,30,3,439,1,10,0,0,30;\nAA;\nCN,30,3,443,1,10,0,0,30;\nAA;\nCN,30,3,447,1,10,0,0,30;\nAA;\nCN,30,3,451,1,10,0,0,30;\nAA;\nCN,30,3,456,1,10,0,0,30;\nAA;\nCN,30,3,461,1,10,0,0,30;\nAA;\nCN,30,3,466,1,10,0,0,30;\nAA;\nCN,30,3,471,1,10,0,0,30;\nAA;\nCN,30,3,476,1,10,0,0,30;\nAA;\nCN,30,3,481,1,10,0,0,30;\nAA;\nCN,30,3,486,1,10,0,0,30;\nAA;\nCN,30,3,491,1,10,0,0,30;\nAA;\nCN,30,3,496,1,10,0,0,30;\nAA;\nCN,30,3,501,1,10,0,0,30;\nAA;\nCN,30,3,506,1,10,0,0,30;\nAA;\nCN,30,3,511,1,10,0,0,30;\nAA;\nCN,30,3,516,1,10,0,0,30;\nAA;\nCN,30,3,521,1,10,0,0,30;\nAA;\nCN,30,3,526,1,10,0,0,30;\nAA;\nCN,30,3,531,1,10,0,0,30;\nAA;\nCN,30,3,536,1,10,0,0,30;\nAA;\nCN,30,3,541,1,10,0,0,30;\nAA;\nCN,30,3,546,1,10,0,0,30;\nAA;\nCN,30,3,551,1,10,0,0,30;\nAA;\nCN,30,3,557,1,10,0,0,30;\nAA;\nCN,30,3,563,1,10,0,0,30;\nAA;\nCN,30,3,569,1,10,0,0,30;\nAA;\nCN,30,3,575,1,10,0,0,30;\nAA;\nCN,30,3,581,1,10,0,0,30;\nAA;\nCN,30,3,587,1,10,0,0,30;\nAA;\nCN,30,3,593,1,10,0,0,30;\nAA;\nCN,30,3,599,1,10,0,0,30;\nAA;\nCN,30,3,605,1,10,0,0,30;\nAA;\nCN,30,3,611,1,10,0,0,30;\nAA;\nCN,30,3,617,1,10,0,0,30;\nAA;\nCN,30,3,623,1,10,0,0,30;\nAA;\nCN,30,3,629,1,10,0,0,30;\nAA;\nCN,30,3,635,1,10,0,0,30;\nAA;\nCN,30,3,641,1,10,0,0,30;\nAA;\nCN,30,3,647,1,10,0,0,30;\nAA;\nCN,30,3,653,1,10,0,0,30;\nAA;\nCN,30,3,660,1,10,0,0,30;\nAA;\nCN,30,3,667,1,10,0,0,30;\nAA;\nCN,30,3,674,1,10,0,0,30;\nAA;\nCN,30,3,681,1,10,0,0,30;\nAA;\nCN,30,3,688,1,10,0,0,30;\nAA;\nCN,30,3,695,1,10,0,0,30;\nAA;\nCN,30,3,702,1,10,0,0,30;\nAA;\nCN,30,3,709,1,10,0,0,30;\nAA;\nCN,30,3,716,1,10,0,0,30;\nAA;\nCN,30,3,723,1,10,0,0,30;\nAA;\nCN,30,3,730,1,10,0,0,30;\nAA;\nCN,30,3,737,1,10,0,0,30;\nAA;\nCN,30,3,744,1,10,0,0,30;\nAA;\nCN,30,3,751,1,10,0,0,30;\nAA;\nCN,30,3,759,1,10,0,0,30;\nAA;\nCN,30,3,767,1,10,0,0,30;\nAA;\nCN,30,3,775,1,10,0,0,30;\nAA;\nCN,30,3,783,1,10,0,0,30;\nAA;\nCN,30,3,791,1,10,0,0,30;\nAA;\nCN,30,3,799,1,10,0,0,30;\nAA;\nCN,30,3,807,1,10,0,0,30;\nAA;\nCN,30,3,815,1,10,0,0,30;\nAA;\nCN,30,3,823,1,10,0,0,30;\nAA;\nCN,30,3,831,1,10,0,0,30;\nAA;\nCN,30,3,839,1,10,0,0,30;\nAA;\nCN,30,3,847,1,10,0,0,30;\nAA;\nCN,30,3,855,1,10,0,0,30;\nAA;\nCN,30,3,864,1,10,0,0,30;\nAA;\nCN,30,3,873,1,10,0,0,30;\nAA;\nCN,30,3,882,1,10,0,0,30;\nAA;\nCN,30,3,891,1,10,0,0,30;\nAA;\nCN,30,3,900,1,10,0,0,30;\nAA;\nCN,30,3,909,1,10,0,0,30;\nAA;\nCN,30,3,918,1,10,0,0,30;\nAA;\nCN,30,3,927,1,10,0,0,30;\nAA;\nCN,30,3,936,1,10,0,0,30;\nAA;\nCN,30,3,945,1,10,0,0,30;\nAA;\nCN,30,3,954,1,10,0,0,30;\nAA;\nCN,30,3,964,1,10,0,0,30;\nAA;\nCN,30,3,974,1,10,0,0,30;\nAA;\nCN,30,3,984,1,10,0,0,30;\nAA;\nCN,30,3,994,1,10,0,0,30;\nAA;\nCN,30,3,1004,1,10,0,0,30;\nAA;\nCN,30,3,1014,1,10,0,0,30;\nAA;\nCN,30,3,1024,1,10,0,0,30;\nAA;\nCN,30,3,1034,1,10,0,0,30;\nAA;\nCN,30,3,1044,1,10,0,0,30;\nAA;\nCN,30,3,1054,1,10,0,0,30;\nAA;\nCN,30,3,1065,1,10,0,0,30;\nAA;\nCN,30,3,1076,1,10,0,0,30;\nAA;\nCN,30,3,1087,1,10,0,0,30;\nAA;\nCN,30,3,1098,1,10,0,0,30;\nAA;\nCN,30,3,1109,1,10,0,0,30;\nAA;\nCN,30,3,1120,1,10,0,0,30;\nAA;\nCN,30,3,1131,1,10,0,0,30;\nAA;\nCN,30,3,1142,1,10,0,0,30;\nAA;\nCN,30,3,1153,1,10,0,0,30;\nAA;\nCN,30,3,1165,1,10,0,0,30;\nAA;\nCN,30,3,1177,1,10,0,0,30;\nAA;\nCN,30,3,1189,1,10,0,0,30;\nAA;\nCN,30,3,1201,1,10,0,0,30;\nAA;\nCN,30,3,1213,1,10,0,0,30;\nAA;\nCN,30,3,1225,1,10,0,0,30;\nAA;\nCN,30,3,1237,1,10,0,0,30;\nAA;\nCN,30,3,1249,1,10,0,0,30;\nAA;\nCN,30,3,1261,1,10,0,0,30;\nAA;\nCN,30,3,1274,1,10,0,0,30;\nAA;\nCN,30,3,1287,1,10,0,0,30;\nAA;\nCN,30,3,1300,1,10,0,0,30;\nAA;\nCN,30,3,1313,1,10,0,0,30;\nAA;\nCN,30,3,1326,1,10,0,0,30;\nAA;\nCN,30,3,1339,1,10,0,0,30;\nAA;\nCN,30,3,1352,1,10,0,0,30;\nAA;\nCN,30,3,1366,1,10,0,0,30;\nAA;\nCN,30,3,1380,1,10,0,0,30;\nAA;\nCN,30,3,1394,1,10,0,0,30;\nAA;\nCN,30,3,1408,1,10,0,0,30;\nAA;\nCN,30,3,1422,1,10,0,0,30;\nAA;\nCN,30,3,1436,1,10,0,0,30;\nAA;\nCN,30,3,1450,1,10,0,0,30;\nAA;\nCN,30,3,1464,1,10,0,0,30;\nAA;\nCN,30,3,1479,1,10,0,0,30;\nAA;\nCN,30,3,1494,1,10,0,0,30;\nAA;\nCN,30,3,1509,1,10,0,0,30;\nAA;\nCN,30,3,1524,1,10,0,0,30;\nAA;\nCN,30,3,1539,1,10,0,0,30;\nAA;\nCN,30,3,1554,1,10,0,0,30;\nAA;\nCN,30,3,1570,1,10,0,0,30;\nAA;\nCN,30,3,1586,1,10,0,0,30;\nAA;\nCN,30,3,1602,1,10,0,0,30;\nAA;\nCN,30,3,1618,1,10,0,0,30;\nAA;\nCN,30,3,1634,1,10,0,0,30;\nAA;\nCN,30,3,1650,1,10,0,0,30;\nAA;\nCN,30,3,1666,1,10,0,0,30;\nAA;\nCN,30,3,1683,1,10,0,0,30;\nAA;\nCN,30,3,1700,1,10,0,0,30;\nAA;\nCN,30,3,1717,1,10,0,0,30;\nAA;\nCN,30,3,1734,1,10,0,0,30;\nAA;\nCN,30,3,1751,1,10,0,0,30;\nAA;\nCN,30,3,1769,1,10,0,0,30;\nAA;\nCN,30,3,1787,1,10,0,0,30;\nAA;\nCN,30,3,1805,1,10,0,0,30;\nAA;\nCN,30,3,1823,1,10,0,0,30;\nAA;\nCN,30,3,1841,1,10,0,0,30;\nAA;\nCN,30,3,1859,1,10,0,0,30;\nAA;\nCN,30,3,1878,1,10,0,0,30;\nAA;\nCN,30,3,1897,1,10,0,0,30;\nAA;\nCN,30,3,1916,1,10,0,0,30;\nAA;\nCN,30,3,1935,1,10,0,0,30;\nAA;\nCN,30,3,1954,1,10,0,0,30;\nAA;\nCN,30,3,1974,1,10,0,0,30;\nAA;\nCN,30,3,1994,1,10,0,0,30;\nAA;\nCN,30,3,2014,1,10,0,0,30;\nAA;\nCN,30,3,2034,1,10,0,0,30;\nAA;\nCN,30,3,2054,1,10,0,0,30;\nAA;\nCN,30,3,2075,1,10,0,0,30;\nAA;\nCN,30,3,2096,1,10,0,0,30;\nAA;\nCN,30,3,2117,1,10,0,0,30;\nAA;\nCN,30,3,2138,1,10,0,0,30;\nAA;\nCN,30,3,2159,1,10,0,0,30;\nAA;\nCN,30,3,2181,1,10,0,0,30;\nAA;\nCN,30,3,2203,1,10,0,0,30;\nAA;\nCN,30,3,2225,1,10,0,0,30;\nAA;\nCN,30,3,2247,1,10,0,0,30;\nAA;\nCN,30,3,2269,1,10,0,0,30;\nAA;\nCN,30,3,2292,1,10,0,0,30;\nAA;\nCN,30,3,2315,1,10,0,0,30;\nAA;\nCN,30,3,2338,1,10,0,0,30;\nAA;\nCN,30,3,2361,1,10,0,0,30;\nAA;\nCN,30,3,2385,1,10,0,0,30;\nAA;\nCN,30,3,2409,1,10,0,0,30;\nAA;\nCN,30,3,2433,1,10,0,0,30;\nAA;\nCN,30,3,2457,1,10,0,0,30;\nAA;\nCN,30,3,2482,1,10,0,0,30;\nAA;\nCN,30,3,2507,1,10,0,0,30;\nAA;\nCN,30,3,2532,1,10,0,0,30;\nAA;\nCN,30,3,2557,1,10,0,0,30;\nAA;\nCN,30,3,2583,1,10,0,0,30;\nAA;\nCN,30,3,2609,1,10,0,0,30;\nAA;\nCN,30,3,2635,1,10,0,0,30;\nAA;\nCN,30,3,2661,1,10,0,0,30;\nAA;\nCN,30,3,2688,1,10,0,0,30;\nAA;\nCN,30,3,2715,1,10,0,0,30;\nAA;\nCN,30,3,2742,1,10,0,0,30;\nAA;\nCN,30,3,2769,1,10,0,0,30;\nAA;\nCN,30,3,2797,1,10,0,0,30;\nAA;\nCN,30,3,2825,1,10,0,0,30;\nAA;\nCN,30,3,2853,1,10,0,0,30;\nAA;\nCN,30,3,2882,1,10,0,0,30;\nAA;\nCN,30,3,2911,1,10,0,0,30;\nAA;\nCN,30,3,2940,1,10,0,0,30;\nAA;\nCN,30,3,2969,1,10,0,0,30;\nAA;\nCN,30,3,2999,1,10,0,0,30;\nAA;\nCN,30,3,3029,1,10,0,0,30;\nAA;\nCN,30,3,3059,1,10,0,0,30;\nAA;\nCN,30,3,3090,1,10,0,0,30;\nAA;\nCN,30,3,3121,1,10,0,0,30;\nAA;\nCN,30,3,3152,1,10,0,0,30;\nAA;\nCN,30,3,3184,1,10,0,0,30;\nAA;\nCN,30,3,3216,1,10,0,0,30;\nAA;\nCN,30,3,3248,1,10,0,0,30;\nAA;\nCN,30,3,3280,1,10,0,0,30;\nAA;\nCN,30,3,3313,1,10,0,0,30;\nAA;\nCN,30,3,3346,1,10,0,0,30;\nAA;\nCN,30,3,3379,1,10,0,0,30;\nAA;\nCN,30,3,3413,1,10,0,0,30;\nAA;\nCN,30,3,3447,1,10,0,0,30;\nAA;\nCN,30,3,3481,1,10,0,0,30;\nAA;\nCN,30,3,3516,1,10,0,0,30;\nAA;\nCN,30,3,3551,1,10,0,0,30;\nAA;\nCN,30,3,3587,1,10,0,0,30;\nAA;\nCN,30,3,3623,1,10,0,0,30;\nAA;\nCN,30,3,3659,1,10,0,0,30;\nAA;\nCN,30,3,3696,1,10,0,0,30;\nAA;\nCN,30,3,3733,1,10,0,0,30;\nAA;\nCN,30,3,3770,1,10,0,0,30;\nAA;\nCN,30,3,3808,1,10,0,0,30;\nAA;\nCN,30,3,3846,1,10,0,0,30;\nAA;\nCN,30,3,3884,1,10,0,0,30;\nAA;\nCN,30,3,3923,1,10,0,0,30;\nAA;\nCN,30,3,3962,1,10,0,0,30;\nAA;\nCN,30,3,4002,1,10,0,0,30;\nAA;\nCN,30,3,4042,1,10,0,0,30;\nAA;\nCN,30,3,4082,1,10,0,0,30;\nAA;\nCN,30,3,4123,1,10,0,0,30;\nAA;\nCN,30,3,4164,1,10,0,0,30;\nAA;\nCN,30,3,4206,1,10,0,0,30;\nAA;\nCN,30,3,4248,1,10,0,0,30;\nAA;\nCN,30,3,4290,1,10,0,0,30;\nAA;\nCN,30,3,4333,1,10,0,0,30;\nAA;\nCN,30,3,4376,1,10,0,0,30;\nAA;\nCN,30,3,4420,1,10,0,0,30;\nAA;\nCN,30,3,4464,1,10,0,0,30;\nAA;\nCN,30,3,4509,1,10,0,0,30;\nAA;\nCN,30,3,4554,1,10,0,0,30;\nAA;\nCN,30,3,4600,1,10,0,0,30;\nAA;\nCN,30,3,4646,1,10,0,0,30;\nAA;\nCN,30,3,4692,1,10,0,0,30;\nAA;\nCN,30,3,4739,1,10,0,0,30;\nAA;\nCN,30,3,4786,1,10,0,0,30;\nAA;\nCN,30,3,4834,1,10,0,0,30;\nAA;\nCN,30,3,4882,1,10,0,0,30;\nAA;\nCN,30,3,4931,1,10,0,0,30;\nAA;\nCN,30,3,4980,1,10,0,0,30;\nAA;\nCN,30,3,5030,1,10,0,0,30;\nAA;\nCN,30,3,5080,1,10,0,0,30;\nAA;\nCN,30,3,5131,1,10,0,0,30;\nAA;\nCN,30,3,5182,1,10,0,0,30;\nAA;\nCN,30,3,5234,1,10,0,0,30;\nAA;\nCN,30,3,5286,1,10,0,0,30;\nAA;\nCN,30,3,5339,1,10,0,0,30;\nAA;\nCN,30,3,5392,1,10,0,0,30;\nAA;\nCN,30,3,5446,1,10,0,0,30;\nAA;\nCN,30,3,5500,1,10,0,0,30;\nAA;\nCN,30,3,5555,1,10,0,0,30;\nAA;\nCN,30,3,5611,1,10,0,0,30;\nAA;\nCN,30,3,5667,1,10,0,0,30;\nAA;\nCN,30,3,5724,1,10,0,0,30;\nAA;\nCN,30,3,5781,1,10,0,0,30;\nAA;\nCN,30,3,5839,1,10,0,0,30;\nAA;\nCN,30,3,5897,1,10,0,0,30;\nAA;\nCN,30,3,5956,1,10,0,0,30;\nAA;\nCN,30,3,6016,1,10,0,0,30;\nAA;\nCN,30,3,6076,1,10,0,0,30;\nAA;\nCN,30,3,6137,1,10,0,0,30;\nAA;\nCN,30,3,6198,1,10,0,0,30;\nAA;\nCN,30,3,6260,1,10,0,0,30;\nAA;\nCN,30,3,6323,1,10,0,0,30;\nAA;\nCN,30,3,6386,1,10,0,0,30;\nAA;\nCN,30,3,6450,1,10,0,0,30;\nAA;\nCN,30,3,6514,1,10,0,0,30;\nAA;\nCN,30,3,6579,1,10,0,0,30;\nAA;\nCN,30,3,6645,1,10,0,0,30;\nAA;\nCN,30,3,6711,1,10,0,0,30;\nAA;\nCN,30,3,6778,1,10,0,0,30;\nAA;\nCN,30,3,6846,1,10,0,0,30;\nAA;\nCN,30,3,6914,1,10,0,0,30;\nAA;\nCN,30,3,6983,1,10,0,0,30;\nAA;\nCN,30,3,7053,1,10,0,0,30;\nAA;\nCN,30,3,7124,1,10,0,0,30;\nAA;\nCN,30,3,7195,1,10,0,0,30;\nAA;\nCN,30,3,7267,1,10,0,0,30;\nAA;\nCN,30,3,7340,1,10,0,0,30;\nAA;\nCN,30,3,7413,1,10,0,0,30;\nAA;\nCN,30,3,7487,1,10,0,0,30;\nAA;\nCN,30,3,7562,1,10,0,0,30;\nAA;\nCN,30,3,7638,1,10,0,0,30;\nAA;\nCN,30,3,7714,1,10,0,0,30;\nAA;\nCN,30,3,7791,1,10,0,0,30;\nAA;\nCN,30,3,7869,1,10,0,0,30;\nAA;\nCN,30,3,7948,1,10,0,0,30;\nAA;\nCN,30,3,8027,1,10,0,0,30;\nAA;\nCN,30,3,8107,1,10,0,0,30;\nAA;\nCN,30,3,8188,1,10,0,0,30;\nAA;\nCN,30,3,8270,1,10,0,0,30;\nAA;\nCN,30,3,8353,1,10,0,0,30;\nAA;\nCN,30,3,8437,1,10,0,0,30;\nAA;\nCN,30,3,8521,1,10,0,0,30;\nAA;\nCN,30,3,8606,1,10,0,0,30;\nAA;\nCN,30,3,8692,1,10,0,0,30;\nAA;\nCN,30,3,8779,1,10,0,0,30;\nAA;\nCN,30,3,8867,1,10,0,0,30;\nAA;\nCN,30,3,8956,1,10,0,0,30;\nAA;\nCN,30,3,9046,1,10,0,0,30;\nAA;\nCN,30,3,9136,1,10,0,0,30;\nAA;\nCN,30,3,9227,1,10,0,0,30;\nAA;\nCN,30,3,9319,1,10,0,0,30;\nAA;\nCN,30,3,9412,1,10,0,0,30;\nAA;\nCN,30,3,9506,1,10,0,0,30;\nAA;\nCN,30,3,9601,1,10,0,0,30;\nAA;\nCN,30,3,9697,1,10,0,0,30;\nAA;\nCN,30,3,9794,1,10,0,0,30;\nAA;\nCN,30,3,9892,1,10,0,0,30;\nAA;\nCN,30,3,9991,1,10,0,0,30;\nAA;\nCN,30,3,10091,1,10,0,0,30;\nAA;\nCN,30,3,10192,1,10,0,0,30;\nAA;\nCN,30,3,10294,1,10,0,0,30;\nAA;\nCN,30,3,10397,1,10,0,0,30;\nAA;\nCN,30,3,10501,1,10,0,0,30;\nAA;\nCN,30,3,10606,1,10,0,0,30;\nAA;\nCN,30,3,10712,1,10,0,0,30;\nAA;\nCN,30,3,10819,1,10,0,0,30;\nAA;\nCN,30,3,10927,1,10,0,0,30;\nAA;\nCN,30,3,11036,1,10,0,0,30;\nAA;\nCN,30,3,11146,1,10,0,0,30;\nAA;\nCN,30,3,11257,1,10,0,0,30;\nAA;\nCN,30,3,11370,1,10,0,0,30;\nAA;\nCN,30,3,11484,1,10,0,0,30;\nAA;\nCN,30,3,11599,1,10,0,0,30;\nAA;\nCN,30,3,11715,1,10,0,0,30;\nAA;\nCN,30,3,11832,1,10,0,0,30;\nAA;\nCN,30,3,11950,1,10,0,0,30;\nAA;\nCN,30,3,12070,1,10,0,0,30;\nAA;\nCN,30,3,12191,1,10,0,0,30;\nAA;\nCN,30,3,12313,1,10,0,0,30;\nAA;\nCN,30,3,12436,1,10,0,0,30;\nAA;\nCN,30,3,12560,1,10,0,0,30;\nAA;\nCN,30,3,12686,1,10,0,0,30;\nAA;\nCN,30,3,12813,1,10,0,0,30;\nAA;\nCN,30,3,12941,1,10,0,0,30;\nAA;\nCN,30,3,13070,1,10,0,0,30;\nAA;\nCN,30,3,13201,1,10,0,0,30;\nAA;\nCN,30,3,13333,1,10,0,0,30;\nAA;\nCN,30,3,13466,1,10,0,0,30;\nAA;\nCN,30,3,13601,1,10,0,0,30;\nAA;\nCN,30,3,13737,1,10,0,0,30;\nAA;\nCN,30,3,13874,1,10,0,0,30;\nAA;\nCN,30,3,14013,1,10,0,0,30;\nAA;\nCN,30,3,14153,1,10,0,0,30;\nAA;\nCN,30,3,14295,1,10,0,0,30;\nAA;\nCN,30,3,14438,1,10,0,0,30;\nAA;\nCN,30,3,14582,1,10,0,0,30;\nAA;\nCN,30,3,14728,1,10,0,0,30;\nAA;\nCN,30,3,14875,1,10,0,0,30;\nAA;\nCN,30,3,15024,1,10,0,0,30;\nAA;\nCN,30,3,15174,1,10,0,0,30;\nAA;\nCN,30,3,15326,1,10,0,0,30;\nAA;\nCN,30,3,15479,1,10,0,0,30;\nAA;\nCN,30,3,15634,1,10,0,0,30;\nAA;\nCN,30,3,15790,1,10,0,0,30;\nAA;\nCN,30,3,15948,1,10,0,0,30;\nAA;\nCN,30,3,16107,1,10,0,0,30;\nAA;\nCN,30,3,16268,1,10,0,0,30;\nAA;\nCN,30,3,16431,1,10,0,0,30;\nAA;\nCN,30,3,16595,1,10,0,0,30;\nAA;\nCN,30,3,16761,1,10,0,0,30;\nAA;\nCN,30,3,16929,1,10,0,0,30;\nAA;\nCN,30,3,17098,1,10,0,0,30;\nAA;\nCN,30,3,17269,1,10,0,0,30;\nAA;\nCN,30,3,17442,1,10,0,0,30;\nAA;\nCN,30,3,17616,1,10,0,0,30;\nAA;\nCN,30,3,17792,1,10,0,0,30;\nAA;\nCN,30,3,17970,1,10,0,0,30;\nAA;\nCN,30,3,18150,1,10,0,0,30;\nAA;\nCN,30,3,18332,1,10,0,0,30;\nAA;\nCN,30,3,18515,1,10,0,0,30;\nAA;\nCN,30,3,18700,1,10,0,0,30;\nAA;\nCN,30,3,18887,1,10,0,0,30;\nAA;\nCN,30,3,19076,1,10,0,0,30;\nAA;\nCN,30,3,19267,1,10,0,0,30;\nAA;\nCN,30,3,19460,1,10,0,0,30;\nAA;\nCN,30,3,19655,1,10,0,0,30;\nAA;\nCN,30,3,19852,1,10,0,0,30;\nAA;\nCN,30,3,20051,1,10,0,0,30;\nAA;\nCN,30,3,20252,1,10,0,0,30;\nAA;\nCN,30,3,20455,1,10,0,0,30;\nAA;\nCN,30,3,20660,1,10,0,0,30;\nAA;\nCN,30,3,20867,1,10,0,0,30;\nAA;\nCN,30,3,21076,1,10,0,0,30;\nAA;\nCN,30,3,21287,1,10,0,0,30;\nAA;\nCN,30,3,21500,1,10,0,0,30;\nAA;\nCN,30,3,21715,1,10,0,0,30;\nAA;\nCN,30,3,21932,1,10,0,0,30;\nAA;\nCN,30,3,22151,1,10,0,0,30;\nAA;\nCN,30,3,22373,1,10,0,0,30;\nAA;\nCN,30,3,22597,1,10,0,0,30;\nAA;\nCN,30,3,22823,1,10,0,0,30;\nAA;\nCN,30,3,23051,1,10,0,0,30;\nAA;\nCN,30,3,23282,1,10,0,0,30;\nAA;\nCN,30,3,23515,1,10,0,0,30;\nAA;\nCN,30,3,23750,1,10,0,0,30;\nAA;\nCN,30,3,23988,1,10,0,0,30;\nAA;\nCN,30,3,24228,1,10,0,0,30;\nAA;\nCN,30,3,24470,1,10,0,0,30;\nAA;\nCN,30,3,24715,1,10,0,0,30;\nAA;\nCN,30,3,24962,1,10,0,0,30;\nAA;\nCN,30,3,25212,1,10,0,0,30;\nAA;\nCN,30,3,25464,1,10,0,0,30;\nAA;\nCN,30,3,25719,1,10,0,0,30;\nAA;\nCN,30,3,25976,1,10,0,0,30;\nAA;\nCN,30,3,26236,1,10,0,0,30;\nAA;\nCN,30,3,26498,1,10,0,0,30;\nAA;\nCN,30,3,26763,1,10,0,0,30;\nAA;\nCN,30,3,27031,1,10,0,0,30;\nAA;\nCN,30,3,27301,1,10,0,0,30;\nAA;\nCN,30,3,27574,1,10,0,0,30;\nAA;\nCN,30,3,27850,1,10,0,0,30;\nAA;\nCN,30,3,28128,1,10,0,0,30;\nAA;\nCN,30,3,28409,1,10,0,0,30;\nAA;\nCN,30,3,28693,1,10,0,0,30;\nAA;\nCN,30,3,28980,1,10,0,0,30;\nAA;\nCN,30,3,29270,1,10,0,0,30;\nAA;\nCN,30,3,29563,1,10,0,0,30;\nAA;\nCN,30,3,29859,1,10,0,0,30;\nAA;\nCN,30,3,30158,1,10,0,0,30;\nAA;\nCN,30,3,30460,1,10,0,0,30;\nAA;\nCN,30,3,30765,1,10,0,0,30;\nAA;\nCN,30,3,31073,1,10,0,0,30;\nAA;\nCN,30,3,31384,1,10,0,0,30;\nAA;\nCN,30,3,31698,1,10,0,0,30;\nAA;\nCN,30,3,32015,1,10,0,0,30;\nAA;\nCN,30,3,32335,1,10,0,0,30;\nAA;\nCN,30,3,32658,1,10,0,0,30;\nAA;\nCN,30,3,32985,1,10,0,0,30;\nAA;\nCN,30,3,33315,1,10,0,0,30;\nAA;\nCN,30,3,33648,1,10,0,0,30;\nAA;\nCN,30,3,33984,1,10,0,0,30;\nAA;\nCN,30,3,34324,1,10,0,0,30;\nAA;\nCN,30,3,34667,1,10,0,0,30;\nAA;\nCN,30,3,35014,1,10,0,0,30;\nAA;\nCN,30,3,35364,1,10,0,0,30;\nAA;\nCN,30,3,35718,1,10,0,0,30;\nAA;\nCN,30,3,36075,1,10,0,0,30;\nAA;\nCN,30,3,36436,1,10,0,0,30;\nAA;\nCN,30,3,36800,1,10,0,0,30;\nAA;\nCN,30,3,37168,1,10,0,0,30;\nAA;\nCN,30,3,37540,1,10,0,0,30;\nAA;\nCN,30,3,37915,1,10,0,0,30;\nAA;\nCN,30,3,38294,1,10,0,0,30;\nAA;\nCN,30,3,38677,1,10,0,0,30;\nAA;\nCN,30,3,39064,1,10,0,0,30;\nAA;\nCN,30,3,39455,1,10,0,0,30;\nAA;\nCN,30,3,39850,1,10,0,0,30;\nAA;\nCN,30,3,40248,1,10,0,0,30;\nAA;\nCN,30,3,40650,1,10,0,0,30;\nAA;\nCN,30,3,41056,1,10,0,0,30;\nAA;\nCN,30,3,41467,1,10,0,0,30;\nAA;\nCN,30,3,41882,1,10,0,0,30;\nAA;\nCN,30,3,42301,1,10,0,0,30;\nAA;\nCN,30,3,42724,1,10,0,0,30;\nAA;\nCN,30,3,43151,1,10,0,0,30;\nAA;\nCN,30,3,43583,1,10,0,0,30;\nAA;\nCN,30,3,44019,1,10,0,0,30;\nAA;\nCN,30,3,44459,1,10,0,0,30;\nAA;\nCN,30,3,44904,1,10,0,0,30;\nAA;\nCN,30,3,45353,1,10,0,0,30;\nAA;\nCN,30,3,45807,1,10,0,0,30;\nAA;\nCN,30,3,46265,1,10,0,0,30;\nAA;\nCN,30,3,46728,1,10,0,0,30;\nAA;\nCN,30,3,47195,1,10,0,0,30;\nAA;\nCN,30,3,47667,1,10,0,0,30;\nAA;\nCN,30,3,48144,1,10,0,0,30;\nAA;\nCN,30,3,48625,1,10,0,0,30;\nAA;\nCN,30,3,49111,1,10,0,0,30;\nAA;\nCN,30,3,49602,1,10,0,0,30;\nAA;\nCN,30,3,50098,1,10,0,0,30;\nAA;\nCN,30,3,50599,1,10,0,0,30;\nAA;\nCN,30,3,51105,1,10,0,0,30;\nAA;\nCN,30,3,51616,1,10,0,0,30;\nAA;\nCN,30,3,52132,1,10,0,0,30;\nAA;\nCN,30,3,52653,1,10,0,0,30;\nAA;\nCN,30,3,53180,1,10,0,0,30;\nAA;\nCN,30,3,53712,1,10,0,0,30;\nAA;\nCN,30,3,54249,1,10,0,0,30;\nAA;\nCN,30,3,54791,1,10,0,0,30;\nAA;\nCN,30,3,55339,1,10,0,0,30;\nAA;\nCN,30,3,55892,1,10,0,0,30;\nAA;\nCN,30,3,56451,1,10,0,0,30;\nAA;\nCN,30,3,57016,1,10,0,0,30;\nAA;\nCN,30,3,57586,1,10,0,0,30;\nAA;\nCN,30,3,58162,1,10,0,0,30;\nAA;\nCN,30,3,58744,1,10,0,0,30;\nAA;\nCN,30,3,59331,1,10,0,0,30;\nAA;\nCN,30,3,59924,1,10,0,0,30;\nAA;\nCN,30,3,60523,1,10,0,0,30;\nAA;\nCN,30,3,61128,1,10,0,0,30;\nAA;\nCN,30,3,61739,1,10,0,0,30;\nAA;\nCN,30,3,62356,1,10,0,0,30;\nAA;\nCN,30,3,62980,1,10,0,0,30;\nAA;\nCN,30,3,63610,1,10,0,0,30;\nAA;\nCN,30,3,64246,1,10,0,0,30;\nAA;\nCN,30,3,64888,1,10,0,0,30;\nAA;\nCN,30,3,65537,1,10,0,0,30;\nAA;\nCN,30,3,66192,1,10,0,0,30;\nAA;\nCN,30,3,66854,1,10,0,0,30;\nAA;\nCN,30,3,67523,1,10,0,0,30;\nAA;\nCN,30,3,68198,1,10,0,0,30;\nAA;\nCN,30,3,68880,1,10,0,0,30;\nAA;\nCN,30,3,69569,1,10,0,0,30;\nAA;\nCN,30,3,70265,1,10,0,0,30;\nAA;\nCN,30,3,70968,1,10,0,0,30;\nAA;\nCN,30,3,71678,1,10,0,0,30;\nAA;\nCN,30,3,72395,1,10,0,0,30;\nAA;\nCN,30,3,73119,1,10,0,0,30;\nAA;\nCN,30,3,73850,1,10,0,0,30;\nAA;\nCN,30,3,74588,1,10,0,0,30;\nAA;\nCN,30,3,75334,1,10,0,0,30;\nAA;\nCN,30,3,76087,1,10,0,0,30;\nAA;\nCN,30,3,76848,1,10,0,0,30;\nAA;\nCN,30,3,77616,1,10,0,0,30;\nAA;\nCN,30,3,78392,1,10,0,0,30;\nAA;\nCN,30,3,79176,1,10,0,0,30;\nAA;\nCN,30,3,79968,1,10,0,0,30;\nAA;\nCN,30,3,80000,1,10,0,0,30;\nAA;\nAR;" ("Commandlist")) -> ("outputstring"=w8:string)  [unwired: 10 in]
      n18 = call-dynamic "set wait.vi"("error in (no error)"=w33, "wait"=i32[] [1200], "TestInterface in"=w34) -> ("error out"=w5:errorcluster, "TestInterface out"=w32:refnum<class "HF-Felder.lvclass">)  [unwired: 7 in]
      n19 = call-dynamic "set Commandlist.vi"("error in (no error)"=w5, "Commandlist"=w8, "TestInterface (Eingang)"=w32) -> ("error out"=w47:errorcluster, "TestInterface (Ausgang)"=w64:refnum<class "HF-Felder.lvclass">)  [unwired: 7 in]
      n20 = call-dynamic "set name.vi"("error in (no error)"=w47, "name"="Standardtest: HF-Felder 1s,1V,150kHz - 80MHz,80% Amod 1kHz", "TestInterface (Eingang)"=refnum<class "HF-Felder.lvclass"> refnum ("HF-Felder.lvclass")) -> ("error out"=w83:errorcluster, "TestInterface (Ausgang)"=w80:refnum<class "HF-Felder.lvclass">)  [unwired: 7 in]
      n21 = call-dynamic "set Command regex.vi"("error in (no error)"=w83, "Command regex"=string[] ["AA"], "TestInterface (Eingang)"=w80) -> ("error out"=w16:errorcluster, "TestInterface (Ausgang)"=w15:refnum<class "HF-Felder.lvclass">)  [unwired: 7 in]
      n22 = call-dynamic "set parameter table.vi"("error in (no error)"=w16, "parameter table"=string[][] [["Amplitude", "1V"], ["Frequenzbereich", "150kHz bis 80MHz"], ["Modulationsart", "Amplitudenmodulation"], ["Modulationsfrequenz", "1kHz"], ["Schrittweite", "< 1%"], ["Beeinflussungszeit je Schritt", "1s"], ["gefordertes Bewertungskriterium", "A"], ["erreichtes Bewertungskriterium", ""]] ("parameters"), "TestInterface in"=w15) -> ("error out"=w13:errorcluster, "TestInterface out"=w12:refnum<class "HF-Felder.lvclass">)  [unwired: 7 in]
      n23 = call-dynamic "set Parameters.vi"("error in (no error)"=w13, "parameters"=string[] ["1", "150", "8000", "1", "3"], "TestInterface (Eingang)"=w12) -> ("error out"=w84:errorcluster, "TestInterface (Ausgang)"=w81:refnum<class "HF-Felder.lvclass">)  [unwired: 7 in]
      n24 = call-dynamic "set response.vi"("error in (no error)"=w84, "response?"=bool[] [TRUE], "TestInterface (Eingang)"=w81) -> ("error out"=w85:errorcluster, "TestInterface (Ausgang)"=w82:refnum<class "HF-Felder.lvclass">)  [unwired: 7 in]
      n25 = call-dynamic "set timings.vi"("error in (no error)"=w85, "timings"=i32[] [1200, 1200], "TestInterface (Eingang)"=w82) -> ("error out"=w42:errorcluster, "TestInterface (Ausgang)"=w43:refnum<class "HF-Felder.lvclass">)  [unwired: 7 in]
      n26 = call "discardCommandsWithBadChecksum.vi"("multi-line string"="*rst\nCC;\nBW;\nBS,1;\n*rst\nCN,10,3,150,1,10,0,0,10;\nAA;\nCN,10,3,152,1,10,0,0,10;\nAA;\nCN,10,3,154,1,10,0,0,10;\nAA;\nCN,10,3,156,1,10,0,0,10;\nAA;\nCN,10,3,158,1,10,0,0,10;\nAA;\nCN,10,3,160,1,10,0,0,10;\nAA;\nCN,10,3,162,1,10,0,0,10;\nAA;\nCN,10,3,164,1,10,0,0,10;\nAA;\nCN,10,3,166,1,10,0,0,10;\nAA;\nCN,10,3,168,1,10,0,0,10;\nAA;\nCN,10,3,170,1,10,0,0,10;\nAA;\nCN,10,3,172,1,10,0,0,10;\nAA;\nCN,10,3,174,1,10,0,0,10;\nAA;\nCN,10,3,176,1,10,0,0,10;\nAA;\nCN,10,3,178,1,10,0,0,10;\nAA;\nCN,10,3,180,1,10,0,0,10;\nAA;\nCN,10,3,182,1,10,0,0,10;\nAA;\nCN,10,3,184,1,10,0,0,10;\nAA;\nCN,10,3,186,1,10,0,0,10;\nAA;\nCN,10,3,188,1,10,0,0,10;\nAA;\nCN,10,3,190,1,10,0,0,10;\nAA;\nCN,10,3,192,1,10,0,0,10;\nAA;\nCN,10,3,194,1,10,0,0,10;\nAA;\nCN,10,3,196,1,10,0,0,10;\nAA;\nCN,10,3,198,1,10,0,0,10;\nAA;\nCN,10,3,200,1,10,0,0,10;\nAA;\nCN,10,3,202,1,10,0,0,10;\nAA;\nCN,10,3,204,1,10,0,0,10;\nAA;\nCN,10,3,206,1,10,0,0,10;\nAA;\nCN,10,3,208,1,10,0,0,10;\nAA;\nCN,10,3,210,1,10,0,0,10;\nAA;\nCN,10,3,212,1,10,0,0,10;\nAA;\nCN,10,3,214,1,10,0,0,10;\nAA;\nCN,10,3,216,1,10,0,0,10;\nAA;\nCN,10,3,218,1,10,0,0,10;\nAA;\nCN,10,3,220,1,10,0,0,10;\nAA;\nCN,10,3,222,1,10,0,0,10;\nAA;\nCN,10,3,224,1,10,0,0,10;\nAA;\nCN,10,3,226,1,10,0,0,10;\nAA;\nCN,10,3,228,1,10,0,0,10;\nAA;\nCN,10,3,230,1,10,0,0,10;\nAA;\nCN,10,3,232,1,10,0,0,10;\nAA;\nCN,10,3,234,1,10,0,0,10;\nAA;\nCN,10,3,236,1,10,0,0,10;\nAA;\nCN,10,3,238,1,10,0,0,10;\nAA;\nCN,10,3,240,1,10,0,0,10;\nAA;\nCN,10,3,242,1,10,0,0,10;\nAA;\nCN,10,3,244,1,10,0,0,10;\nAA;\nCN,10,3,246,1,10,0,0,10;\nAA;\nCN,10,3,248,1,10,0,0,10;\nAA;\nCN,10,3,250,1,10,0,0,10;\nAA;\nCN,10,3,252,1,10,0,0,10;\nAA;\nCN,10,3,255,1,10,0,0,10;\nAA;\nCN,10,3,258,1,10,0,0,10;\nAA;\nCN,10,3,261,1,10,0,0,10;\nAA;\nCN,10,3,264,1,10,0,0,10;\nAA;\nCN,10,3,267,1,10,0,0,10;\nAA;\nCN,10,3,270,1,10,0,0,10;\nAA;\nCN,10,3,273,1,10,0,0,10;\nAA;\nCN,10,3,276,1,10,0,0,10;\nAA;\nCN,10,3,279,1,10,0,0,10;\nAA;\nCN,10,3,282,1,10,0,0,10;\nAA;\nCN,10,3,285,1,10,0,0,10;\nAA;\nCN,10,3,288,1,10,0,0,10;\nAA;\nCN,10,3,291,1,10,0,0,10;\nAA;\nCN,10,3,294,1,10,0,0,10;\nAA;\nCN,10,3,297,1,10,0,0,10;\nAA;\nCN,10,3,300,1,10,0,0,10;\nAA;\nCN,10,3,303,1,10,0,0,10;\nAA;\nCN,10,3,306,1,10,0,0,10;\nAA;\nCN,10,3,309,1,10,0,0,10;\nAA;\nCN,10,3,312,1,10,0,0,10;\nAA;\nCN,10,3,315,1,10,0,0,10;\nAA;\nCN,10,3,318,1,10,0,0,10;\nAA;\nCN,10,3,321,1,10,0,0,10;\nAA;\nCN,10,3,324,1,10,0,0,10;\nAA;\nCN,10,3,327,1,10,0,0,10;\nAA;\nCN,10,3,330,1,10,0,0,10;\nAA;\nCN,10,3,333,1,10,0,0,10;\nAA;\nCN,10,3,336,1,10,0,0,10;\nAA;\nCN,10,3,339,1,10,0,0,10;\nAA;\nCN,10,3,342,1,10,0,0,10;\nAA;\nCN,10,3,345,1,10,0,0,10;\nAA;\nCN,10,3,348,1,10,0,0,10;\nAA;\nCN,10,3,351,1,10,0,0,10;\nAA;\nCN,10,3,355,1,10,0,0,10;\nAA;\nCN,10,3,359,1,10,0,0,10;\nAA;\nCN,10,3,363,1,10,0,0,10;\nAA;\nCN,10,3,367,1,10,0,0,10;\nAA;\nCN,10,3,371,1,10,0,0,10;\nAA;\nCN,10,3,375,1,10,0,0,10;\nAA;\nCN,10,3,379,1,10,0,0,10;\nAA;\nCN,10,3,383,1,10,0,0,10;\nAA;\nCN,10,3,387,1,10,0,0,10;\nAA;\nCN,10,3,391,1,10,0,0,10;\nAA;\nCN,10,3,395,1,10,0,0,10;\nAA;\nCN,10,3,399,1,10,0,0,10;\nAA;\nCN,10,3,403,1,10,0,0,10;\nAA;\nCN,10,3,407,1,10,0,0,10;\nAA;\nCN,10,3,411,1,10,0,0,10;\nAA;\nCN,10,3,415,1,10,0,0,10;\nAA;\nCN,10,3,419,1,10,0,0,10;\nAA;\nCN,10,3,423,1,10,0,0,10;\nAA;\nCN,10,3,427,1,10,0,0,10;\nAA;\nCN,10,3,431,1,10,0,0,10;\nAA;\nCN,10,3,435,1,10,0,0,10;\nAA;\nCN,10,3,439,1,10,0,0,10;\nAA;\nCN,10,3,443,1,10,0,0,10;\nAA;\nCN,10,3,447,1,10,0,0,10;\nAA;\nCN,10,3,451,1,10,0,0,10;\nAA;\nCN,10,3,456,1,10,0,0,10;\nAA;\nCN,10,3,461,1,10,0,0,10;\nAA;\nCN,10,3,466,1,10,0,0,10;\nAA;\nCN,10,3,471,1,10,0,0,10;\nAA;\nCN,10,3,476,1,10,0,0,10;\nAA;\nCN,10,3,481,1,10,0,0,10;\nAA;\nCN,10,3,486,1,10,0,0,10;\nAA;\nCN,10,3,491,1,10,0,0,10;\nAA;\nCN,10,3,496,1,10,0,0,10;\nAA;\nCN,10,3,501,1,10,0,0,10;\nAA;\nCN,10,3,506,1,10,0,0,10;\nAA;\nCN,10,3,511,1,10,0,0,10;\nAA;\nCN,10,3,516,1,10,0,0,10;\nAA;\nCN,10,3,521,1,10,0,0,10;\nAA;\nCN,10,3,526,1,10,0,0,10;\nAA;\nCN,10,3,531,1,10,0,0,10;\nAA;\nCN,10,3,536,1,10,0,0,10;\nAA;\nCN,10,3,541,1,10,0,0,10;\nAA;\nCN,10,3,546,1,10,0,0,10;\nAA;\nCN,10,3,551,1,10,0,0,10;\nAA;\nCN,10,3,557,1,10,0,0,10;\nAA;\nCN,10,3,563,1,10,0,0,10;\nAA;\nCN,10,3,569,1,10,0,0,10;\nAA;\nCN,10,3,575,1,10,0,0,10;\nAA;\nCN,10,3,581,1,10,0,0,10;\nAA;\nCN,10,3,587,1,10,0,0,10;\nAA;\nCN,10,3,593,1,10,0,0,10;\nAA;\nCN,10,3,599,1,10,0,0,10;\nAA;\nCN,10,3,605,1,10,0,0,10;\nAA;\nCN,10,3,611,1,10,0,0,10;\nAA;\nCN,10,3,617,1,10,0,0,10;\nAA;\nCN,10,3,623,1,10,0,0,10;\nAA;\nCN,10,3,629,1,10,0,0,10;\nAA;\nCN,10,3,635,1,10,0,0,10;\nAA;\nCN,10,3,641,1,10,0,0,10;\nAA;\nCN,10,3,647,1,10,0,0,10;\nAA;\nCN,10,3,653,1,10,0,0,10;\nAA;\nCN,10,3,660,1,10,0,0,10;\nAA;\nCN,10,3,667,1,10,0,0,10;\nAA;\nCN,10,3,674,1,10,0,0,10;\nAA;\nCN,10,3,681,1,10,0,0,10;\nAA;\nCN,10,3,688,1,10,0,0,10;\nAA;\nCN,10,3,695,1,10,0,0,10;\nAA;\nCN,10,3,702,1,10,0,0,10;\nAA;\nCN,10,3,709,1,10,0,0,10;\nAA;\nCN,10,3,716,1,10,0,0,10;\nAA;\nCN,10,3,723,1,10,0,0,10;\nAA;\nCN,10,3,730,1,10,0,0,10;\nAA;\nCN,10,3,737,1,10,0,0,10;\nAA;\nCN,10,3,744,1,10,0,0,10;\nAA;\nCN,10,3,751,1,10,0,0,10;\nAA;\nCN,10,3,759,1,10,0,0,10;\nAA;\nCN,10,3,767,1,10,0,0,10;\nAA;\nCN,10,3,775,1,10,0,0,10;\nAA;\nCN,10,3,783,1,10,0,0,10;\nAA;\nCN,10,3,791,1,10,0,0,10;\nAA;\nCN,10,3,799,1,10,0,0,10;\nAA;\nCN,10,3,807,1,10,0,0,10;\nAA;\nCN,10,3,815,1,10,0,0,10;\nAA;\nCN,10,3,823,1,10,0,0,10;\nAA;\nCN,10,3,831,1,10,0,0,10;\nAA;\nCN,10,3,839,1,10,0,0,10;\nAA;\nCN,10,3,847,1,10,0,0,10;\nAA;\nCN,10,3,855,1,10,0,0,10;\nAA;\nCN,10,3,864,1,10,0,0,10;\nAA;\nCN,10,3,873,1,10,0,0,10;\nAA;\nCN,10,3,882,1,10,0,0,10;\nAA;\nCN,10,3,891,1,10,0,0,10;\nAA;\nCN,10,3,900,1,10,0,0,10;\nAA;\nCN,10,3,909,1,10,0,0,10;\nAA;\nCN,10,3,918,1,10,0,0,10;\nAA;\nCN,10,3,927,1,10,0,0,10;\nAA;\nCN,10,3,936,1,10,0,0,10;\nAA;\nCN,10,3,945,1,10,0,0,10;\nAA;\nCN,10,3,954,1,10,0,0,10;\nAA;\nCN,10,3,964,1,10,0,0,10;\nAA;\nCN,10,3,974,1,10,0,0,10;\nAA;\nCN,10,3,984,1,10,0,0,10;\nAA;\nCN,10,3,994,1,10,0,0,10;\nAA;\nCN,10,3,1004,1,10,0,0,10;\nAA;\nCN,10,3,1014,1,10,0,0,10;\nAA;\nCN,10,3,1024,1,10,0,0,10;\nAA;\nCN,10,3,1034,1,10,0,0,10;\nAA;\nCN,10,3,1044,1,10,0,0,10;\nAA;\nCN,10,3,1054,1,10,0,0,10;\nAA;\nCN,10,3,1065,1,10,0,0,10;\nAA;\nCN,10,3,1076,1,10,0,0,10;\nAA;\nCN,10,3,1087,1,10,0,0,10;\nAA;\nCN,10,3,1098,1,10,0,0,10;\nAA;\nCN,10,3,1109,1,10,0,0,10;\nAA;\nCN,10,3,1120,1,10,0,0,10;\nAA;\nCN,10,3,1131,1,10,0,0,10;\nAA;\nCN,10,3,1142,1,10,0,0,10;\nAA;\nCN,10,3,1153,1,10,0,0,10;\nAA;\nCN,10,3,1165,1,10,0,0,10;\nAA;\nCN,10,3,1177,1,10,0,0,10;\nAA;\nCN,10,3,1189,1,10,0,0,10;\nAA;\nCN,10,3,1201,1,10,0,0,10;\nAA;\nCN,10,3,1213,1,10,0,0,10;\nAA;\nCN,10,3,1225,1,10,0,0,10;\nAA;\nCN,10,3,1237,1,10,0,0,10;\nAA;\nCN,10,3,1249,1,10,0,0,10;\nAA;\nCN,10,3,1261,1,10,0,0,10;\nAA;\nCN,10,3,1274,1,10,0,0,10;\nAA;\nCN,10,3,1287,1,10,0,0,10;\nAA;\nCN,10,3,1300,1,10,0,0,10;\nAA;\nCN,10,3,1313,1,10,0,0,10;\nAA;\nCN,10,3,1326,1,10,0,0,10;\nAA;\nCN,10,3,1339,1,10,0,0,10;\nAA;\nCN,10,3,1352,1,10,0,0,10;\nAA;\nCN,10,3,1366,1,10,0,0,10;\nAA;\nCN,10,3,1380,1,10,0,0,10;\nAA;\nCN,10,3,1394,1,10,0,0,10;\nAA;\nCN,10,3,1408,1,10,0,0,10;\nAA;\nCN,10,3,1422,1,10,0,0,10;\nAA;\nCN,10,3,1436,1,10,0,0,10;\nAA;\nCN,10,3,1450,1,10,0,0,10;\nAA;\nCN,10,3,1464,1,10,0,0,10;\nAA;\nCN,10,3,1479,1,10,0,0,10;\nAA;\nCN,10,3,1494,1,10,0,0,10;\nAA;\nCN,10,3,1509,1,10,0,0,10;\nAA;\nCN,10,3,1524,1,10,0,0,10;\nAA;\nCN,10,3,1539,1,10,0,0,10;\nAA;\nCN,10,3,1554,1,10,0,0,10;\nAA;\nCN,10,3,1570,1,10,0,0,10;\nAA;\nCN,10,3,1586,1,10,0,0,10;\nAA;\nCN,10,3,1602,1,10,0,0,10;\nAA;\nCN,10,3,1618,1,10,0,0,10;\nAA;\nCN,10,3,1634,1,10,0,0,10;\nAA;\nCN,10,3,1650,1,10,0,0,10;\nAA;\nCN,10,3,1666,1,10,0,0,10;\nAA;\nCN,10,3,1683,1,10,0,0,10;\nAA;\nCN,10,3,1700,1,10,0,0,10;\nAA;\nCN,10,3,1717,1,10,0,0,10;\nAA;\nCN,10,3,1734,1,10,0,0,10;\nAA;\nCN,10,3,1751,1,10,0,0,10;\nAA;\nCN,10,3,1769,1,10,0,0,10;\nAA;\nCN,10,3,1787,1,10,0,0,10;\nAA;\nCN,10,3,1805,1,10,0,0,10;\nAA;\nCN,10,3,1823,1,10,0,0,10;\nAA;\nCN,10,3,1841,1,10,0,0,10;\nAA;\nCN,10,3,1859,1,10,0,0,10;\nAA;\nCN,10,3,1878,1,10,0,0,10;\nAA;\nCN,10,3,1897,1,10,0,0,10;\nAA;\nCN,10,3,1916,1,10,0,0,10;\nAA;\nCN,10,3,1935,1,10,0,0,10;\nAA;\nCN,10,3,1954,1,10,0,0,10;\nAA;\nCN,10,3,1974,1,10,0,0,10;\nAA;\nCN,10,3,1994,1,10,0,0,10;\nAA;\nCN,10,3,2014,1,10,0,0,10;\nAA;\nCN,10,3,2034,1,10,0,0,10;\nAA;\nCN,10,3,2054,1,10,0,0,10;\nAA;\nCN,10,3,2075,1,10,0,0,10;\nAA;\nCN,10,3,2096,1,10,0,0,10;\nAA;\nCN,10,3,2117,1,10,0,0,10;\nAA;\nCN,10,3,2138,1,10,0,0,10;\nAA;\nCN,10,3,2159,1,10,0,0,10;\nAA;\nCN,10,3,2181,1,10,0,0,10;\nAA;\nCN,10,3,2203,1,10,0,0,10;\nAA;\nCN,10,3,2225,1,10,0,0,10;\nAA;\nCN,10,3,2247,1,10,0,0,10;\nAA;\nCN,10,3,2269,1,10,0,0,10;\nAA;\nCN,10,3,2292,1,10,0,0,10;\nAA;\nCN,10,3,2315,1,10,0,0,10;\nAA;\nCN,10,3,2338,1,10,0,0,10;\nAA;\nCN,10,3,2361,1,10,0,0,10;\nAA;\nCN,10,3,2385,1,10,0,0,10;\nAA;\nCN,10,3,2409,1,10,0,0,10;\nAA;\nCN,10,3,2433,1,10,0,0,10;\nAA;\nCN,10,3,2457,1,10,0,0,10;\nAA;\nCN,10,3,2482,1,10,0,0,10;\nAA;\nCN,10,3,2507,1,10,0,0,10;\nAA;\nCN,10,3,2532,1,10,0,0,10;\nAA;\nCN,10,3,2557,1,10,0,0,10;\nAA;\nCN,10,3,2583,1,10,0,0,10;\nAA;\nCN,10,3,2609,1,10,0,0,10;\nAA;\nCN,10,3,2635,1,10,0,0,10;\nAA;\nCN,10,3,2661,1,10,0,0,10;\nAA;\nCN,10,3,2688,1,10,0,0,10;\nAA;\nCN,10,3,2715,1,10,0,0,10;\nAA;\nCN,10,3,2742,1,10,0,0,10;\nAA;\nCN,10,3,2769,1,10,0,0,10;\nAA;\nCN,10,3,2797,1,10,0,0,10;\nAA;\nCN,10,3,2825,1,10,0,0,10;\nAA;\nCN,10,3,2853,1,10,0,0,10;\nAA;\nCN,10,3,2882,1,10,0,0,10;\nAA;\nCN,10,3,2911,1,10,0,0,10;\nAA;\nCN,10,3,2940,1,10,0,0,10;\nAA;\nCN,10,3,2969,1,10,0,0,10;\nAA;\nCN,10,3,2999,1,10,0,0,10;\nAA;\nCN,10,3,3029,1,10,0,0,10;\nAA;\nCN,10,3,3059,1,10,0,0,10;\nAA;\nCN,10,3,3090,1,10,0,0,10;\nAA;\nCN,10,3,3121,1,10,0,0,10;\nAA;\nCN,10,3,3152,1,10,0,0,10;\nAA;\nCN,10,3,3184,1,10,0,0,10;\nAA;\nCN,10,3,3216,1,10,0,0,10;\nAA;\nCN,10,3,3248,1,10,0,0,10;\nAA;\nCN,10,3,3280,1,10,0,0,10;\nAA;\nCN,10,3,3313,1,10,0,0,10;\nAA;\nCN,10,3,3346,1,10,0,0,10;\nAA;\nCN,10,3,3379,1,10,0,0,10;\nAA;\nCN,10,3,3413,1,10,0,0,10;\nAA;\nCN,10,3,3447,1,10,0,0,10;\nAA;\nCN,10,3,3481,1,10,0,0,10;\nAA;\nCN,10,3,3516,1,10,0,0,10;\nAA;\nCN,10,3,3551,1,10,0,0,10;\nAA;\nCN,10,3,3587,1,10,0,0,10;\nAA;\nCN,10,3,3623,1,10,0,0,10;\nAA;\nCN,10,3,3659,1,10,0,0,10;\nAA;\nCN,10,3,3696,1,10,0,0,10;\nAA;\nCN,10,3,3733,1,10,0,0,10;\nAA;\nCN,10,3,3770,1,10,0,0,10;\nAA;\nCN,10,3,3808,1,10,0,0,10;\nAA;\nCN,10,3,3846,1,10,0,0,10;\nAA;\nCN,10,3,3884,1,10,0,0,10;\nAA;\nCN,10,3,3923,1,10,0,0,10;\nAA;\nCN,10,3,3962,1,10,0,0,10;\nAA;\nCN,10,3,4002,1,10,0,0,10;\nAA;\nCN,10,3,4042,1,10,0,0,10;\nAA;\nCN,10,3,4082,1,10,0,0,10;\nAA;\nCN,10,3,4123,1,10,0,0,10;\nAA;\nCN,10,3,4164,1,10,0,0,10;\nAA;\nCN,10,3,4206,1,10,0,0,10;\nAA;\nCN,10,3,4248,1,10,0,0,10;\nAA;\nCN,10,3,4290,1,10,0,0,10;\nAA;\nCN,10,3,4333,1,10,0,0,10;\nAA;\nCN,10,3,4376,1,10,0,0,10;\nAA;\nCN,10,3,4420,1,10,0,0,10;\nAA;\nCN,10,3,4464,1,10,0,0,10;\nAA;\nCN,10,3,4509,1,10,0,0,10;\nAA;\nCN,10,3,4554,1,10,0,0,10;\nAA;\nCN,10,3,4600,1,10,0,0,10;\nAA;\nCN,10,3,4646,1,10,0,0,10;\nAA;\nCN,10,3,4692,1,10,0,0,10;\nAA;\nCN,10,3,4739,1,10,0,0,10;\nAA;\nCN,10,3,4786,1,10,0,0,10;\nAA;\nCN,10,3,4834,1,10,0,0,10;\nAA;\nCN,10,3,4882,1,10,0,0,10;\nAA;\nCN,10,3,4931,1,10,0,0,10;\nAA;\nCN,10,3,4980,1,10,0,0,10;\nAA;\nCN,10,3,5030,1,10,0,0,10;\nAA;\nCN,10,3,5080,1,10,0,0,10;\nAA;\nCN,10,3,5131,1,10,0,0,10;\nAA;\nCN,10,3,5182,1,10,0,0,10;\nAA;\nCN,10,3,5234,1,10,0,0,10;\nAA;\nCN,10,3,5286,1,10,0,0,10;\nAA;\nCN,10,3,5339,1,10,0,0,10;\nAA;\nCN,10,3,5392,1,10,0,0,10;\nAA;\nCN,10,3,5446,1,10,0,0,10;\nAA;\nCN,10,3,5500,1,10,0,0,10;\nAA;\nCN,10,3,5555,1,10,0,0,10;\nAA;\nCN,10,3,5611,1,10,0,0,10;\nAA;\nCN,10,3,5667,1,10,0,0,10;\nAA;\nCN,10,3,5724,1,10,0,0,10;\nAA;\nCN,10,3,5781,1,10,0,0,10;\nAA;\nCN,10,3,5839,1,10,0,0,10;\nAA;\nCN,10,3,5897,1,10,0,0,10;\nAA;\nCN,10,3,5956,1,10,0,0,10;\nAA;\nCN,10,3,6016,1,10,0,0,10;\nAA;\nCN,10,3,6076,1,10,0,0,10;\nAA;\nCN,10,3,6137,1,10,0,0,10;\nAA;\nCN,10,3,6198,1,10,0,0,10;\nAA;\nCN,10,3,6260,1,10,0,0,10;\nAA;\nCN,10,3,6323,1,10,0,0,10;\nAA;\nCN,10,3,6386,1,10,0,0,10;\nAA;\nCN,10,3,6450,1,10,0,0,10;\nAA;\nCN,10,3,6514,1,10,0,0,10;\nAA;\nCN,10,3,6579,1,10,0,0,10;\nAA;\nCN,10,3,6645,1,10,0,0,10;\nAA;\nCN,10,3,6711,1,10,0,0,10;\nAA;\nCN,10,3,6778,1,10,0,0,10;\nAA;\nCN,10,3,6846,1,10,0,0,10;\nAA;\nCN,10,3,6914,1,10,0,0,10;\nAA;\nCN,10,3,6983,1,10,0,0,10;\nAA;\nCN,10,3,7053,1,10,0,0,10;\nAA;\nCN,10,3,7124,1,10,0,0,10;\nAA;\nCN,10,3,7195,1,10,0,0,10;\nAA;\nCN,10,3,7267,1,10,0,0,10;\nAA;\nCN,10,3,7340,1,10,0,0,10;\nAA;\nCN,10,3,7413,1,10,0,0,10;\nAA;\nCN,10,3,7487,1,10,0,0,10;\nAA;\nCN,10,3,7562,1,10,0,0,10;\nAA;\nCN,10,3,7638,1,10,0,0,10;\nAA;\nCN,10,3,7714,1,10,0,0,10;\nAA;\nCN,10,3,7791,1,10,0,0,10;\nAA;\nCN,10,3,7869,1,10,0,0,10;\nAA;\nCN,10,3,7948,1,10,0,0,10;\nAA;\nCN,10,3,8027,1,10,0,0,10;\nAA;\nCN,10,3,8107,1,10,0,0,10;\nAA;\nCN,10,3,8188,1,10,0,0,10;\nAA;\nCN,10,3,8270,1,10,0,0,10;\nAA;\nCN,10,3,8353,1,10,0,0,10;\nAA;\nCN,10,3,8437,1,10,0,0,10;\nAA;\nCN,10,3,8521,1,10,0,0,10;\nAA;\nCN,10,3,8606,1,10,0,0,10;\nAA;\nCN,10,3,8692,1,10,0,0,10;\nAA;\nCN,10,3,8779,1,10,0,0,10;\nAA;\nCN,10,3,8867,1,10,0,0,10;\nAA;\nCN,10,3,8956,1,10,0,0,10;\nAA;\nCN,10,3,9046,1,10,0,0,10;\nAA;\nCN,10,3,9136,1,10,0,0,10;\nAA;\nCN,10,3,9227,1,10,0,0,10;\nAA;\nCN,10,3,9319,1,10,0,0,10;\nAA;\nCN,10,3,9412,1,10,0,0,10;\nAA;\nCN,10,3,9506,1,10,0,0,10;\nAA;\nCN,10,3,9601,1,10,0,0,10;\nAA;\nCN,10,3,9697,1,10,0,0,10;\nAA;\nCN,10,3,9794,1,10,0,0,10;\nAA;\nCN,10,3,9892,1,10,0,0,10;\nAA;\nCN,10,3,9991,1,10,0,0,10;\nAA;\nCN,10,3,10091,1,10,0,0,10;\nAA;\nCN,10,3,10192,1,10,0,0,10;\nAA;\nCN,10,3,10294,1,10,0,0,10;\nAA;\nCN,10,3,10397,1,10,0,0,10;\nAA;\nCN,10,3,10501,1,10,0,0,10;\nAA;\nCN,10,3,10606,1,10,0,0,10;\nAA;\nCN,10,3,10712,1,10,0,0,10;\nAA;\nCN,10,3,10819,1,10,0,0,10;\nAA;\nCN,10,3,10927,1,10,0,0,10;\nAA;\nCN,10,3,11036,1,10,0,0,10;\nAA;\nCN,10,3,11146,1,10,0,0,10;\nAA;\nCN,10,3,11257,1,10,0,0,10;\nAA;\nCN,10,3,11370,1,10,0,0,10;\nAA;\nCN,10,3,11484,1,10,0,0,10;\nAA;\nCN,10,3,11599,1,10,0,0,10;\nAA;\nCN,10,3,11715,1,10,0,0,10;\nAA;\nCN,10,3,11832,1,10,0,0,10;\nAA;\nCN,10,3,11950,1,10,0,0,10;\nAA;\nCN,10,3,12070,1,10,0,0,10;\nAA;\nCN,10,3,12191,1,10,0,0,10;\nAA;\nCN,10,3,12313,1,10,0,0,10;\nAA;\nCN,10,3,12436,1,10,0,0,10;\nAA;\nCN,10,3,12560,1,10,0,0,10;\nAA;\nCN,10,3,12686,1,10,0,0,10;\nAA;\nCN,10,3,12813,1,10,0,0,10;\nAA;\nCN,10,3,12941,1,10,0,0,10;\nAA;\nCN,10,3,13070,1,10,0,0,10;\nAA;\nCN,10,3,13201,1,10,0,0,10;\nAA;\nCN,10,3,13333,1,10,0,0,10;\nAA;\nCN,10,3,13466,1,10,0,0,10;\nAA;\nCN,10,3,13601,1,10,0,0,10;\nAA;\nCN,10,3,13737,1,10,0,0,10;\nAA;\nCN,10,3,13874,1,10,0,0,10;\nAA;\nCN,10,3,14013,1,10,0,0,10;\nAA;\nCN,10,3,14153,1,10,0,0,10;\nAA;\nCN,10,3,14295,1,10,0,0,10;\nAA;\nCN,10,3,14438,1,10,0,0,10;\nAA;\nCN,10,3,14582,1,10,0,0,10;\nAA;\nCN,10,3,14728,1,10,0,0,10;\nAA;\nCN,10,3,14875,1,10,0,0,10;\nAA;\nCN,10,3,15024,1,10,0,0,10;\nAA;\nCN,10,3,15174,1,10,0,0,10;\nAA;\nCN,10,3,15326,1,10,0,0,10;\nAA;\nCN,10,3,15479,1,10,0,0,10;\nAA;\nCN,10,3,15634,1,10,0,0,10;\nAA;\nCN,10,3,15790,1,10,0,0,10;\nAA;\nCN,10,3,15948,1,10,0,0,10;\nAA;\nCN,10,3,16107,1,10,0,0,10;\nAA;\nCN,10,3,16268,1,10,0,0,10;\nAA;\nCN,10,3,16431,1,10,0,0,10;\nAA;\nCN,10,3,16595,1,10,0,0,10;\nAA;\nCN,10,3,16761,1,10,0,0,10;\nAA;\nCN,10,3,16929,1,10,0,0,10;\nAA;\nCN,10,3,17098,1,10,0,0,10;\nAA;\nCN,10,3,17269,1,10,0,0,10;\nAA;\nCN,10,3,17442,1,10,0,0,10;\nAA;\nCN,10,3,17616,1,10,0,0,10;\nAA;\nCN,10,3,17792,1,10,0,0,10;\nAA;\nCN,10,3,17970,1,10,0,0,10;\nAA;\nCN,10,3,18150,1,10,0,0,10;\nAA;\nCN,10,3,18332,1,10,0,0,10;\nAA;\nCN,10,3,18515,1,10,0,0,10;\nAA;\nCN,10,3,18700,1,10,0,0,10;\nAA;\nCN,10,3,18887,1,10,0,0,10;\nAA;\nCN,10,3,19076,1,10,0,0,10;\nAA;\nCN,10,3,19267,1,10,0,0,10;\nAA;\nCN,10,3,19460,1,10,0,0,10;\nAA;\nCN,10,3,19655,1,10,0,0,10;\nAA;\nCN,10,3,19852,1,10,0,0,10;\nAA;\nCN,10,3,20051,1,10,0,0,10;\nAA;\nCN,10,3,20252,1,10,0,0,10;\nAA;\nCN,10,3,20455,1,10,0,0,10;\nAA;\nCN,10,3,20660,1,10,0,0,10;\nAA;\nCN,10,3,20867,1,10,0,0,10;\nAA;\nCN,10,3,21076,1,10,0,0,10;\nAA;\nCN,10,3,21287,1,10,0,0,10;\nAA;\nCN,10,3,21500,1,10,0,0,10;\nAA;\nCN,10,3,21715,1,10,0,0,10;\nAA;\nCN,10,3,21932,1,10,0,0,10;\nAA;\nCN,10,3,22151,1,10,0,0,10;\nAA;\nCN,10,3,22373,1,10,0,0,10;\nAA;\nCN,10,3,22597,1,10,0,0,10;\nAA;\nCN,10,3,22823,1,10,0,0,10;\nAA;\nCN,10,3,23051,1,10,0,0,10;\nAA;\nCN,10,3,23282,1,10,0,0,10;\nAA;\nCN,10,3,23515,1,10,0,0,10;\nAA;\nCN,10,3,23750,1,10,0,0,10;\nAA;\nCN,10,3,23988,1,10,0,0,10;\nAA;\nCN,10,3,24228,1,10,0,0,10;\nAA;\nCN,10,3,24470,1,10,0,0,10;\nAA;\nCN,10,3,24715,1,10,0,0,10;\nAA;\nCN,10,3,24962,1,10,0,0,10;\nAA;\nCN,10,3,25212,1,10,0,0,10;\nAA;\nCN,10,3,25464,1,10,0,0,10;\nAA;\nCN,10,3,25719,1,10,0,0,10;\nAA;\nCN,10,3,25976,1,10,0,0,10;\nAA;\nCN,10,3,26236,1,10,0,0,10;\nAA;\nCN,10,3,26498,1,10,0,0,10;\nAA;\nCN,10,3,26763,1,10,0,0,10;\nAA;\nCN,10,3,27031,1,10,0,0,10;\nAA;\nCN,10,3,27301,1,10,0,0,10;\nAA;\nCN,10,3,27574,1,10,0,0,10;\nAA;\nCN,10,3,27850,1,10,0,0,10;\nAA;\nCN,10,3,28128,1,10,0,0,10;\nAA;\nCN,10,3,28409,1,10,0,0,10;\nAA;\nCN,10,3,28693,1,10,0,0,10;\nAA;\nCN,10,3,28980,1,10,0,0,10;\nAA;\nCN,10,3,29270,1,10,0,0,10;\nAA;\nCN,10,3,29563,1,10,0,0,10;\nAA;\nCN,10,3,29859,1,10,0,0,10;\nAA;\nCN,10,3,30158,1,10,0,0,10;\nAA;\nCN,10,3,30460,1,10,0,0,10;\nAA;\nCN,10,3,30765,1,10,0,0,10;\nAA;\nCN,10,3,31073,1,10,0,0,10;\nAA;\nCN,10,3,31384,1,10,0,0,10;\nAA;\nCN,10,3,31698,1,10,0,0,10;\nAA;\nCN,10,3,32015,1,10,0,0,10;\nAA;\nCN,10,3,32335,1,10,0,0,10;\nAA;\nCN,10,3,32658,1,10,0,0,10;\nAA;\nCN,10,3,32985,1,10,0,0,10;\nAA;\nCN,10,3,33315,1,10,0,0,10;\nAA;\nCN,10,3,33648,1,10,0,0,10;\nAA;\nCN,10,3,33984,1,10,0,0,10;\nAA;\nCN,10,3,34324,1,10,0,0,10;\nAA;\nCN,10,3,34667,1,10,0,0,10;\nAA;\nCN,10,3,35014,1,10,0,0,10;\nAA;\nCN,10,3,35364,1,10,0,0,10;\nAA;\nCN,10,3,35718,1,10,0,0,10;\nAA;\nCN,10,3,36075,1,10,0,0,10;\nAA;\nCN,10,3,36436,1,10,0,0,10;\nAA;\nCN,10,3,36800,1,10,0,0,10;\nAA;\nCN,10,3,37168,1,10,0,0,10;\nAA;\nCN,10,3,37540,1,10,0,0,10;\nAA;\nCN,10,3,37915,1,10,0,0,10;\nAA;\nCN,10,3,38294,1,10,0,0,10;\nAA;\nCN,10,3,38677,1,10,0,0,10;\nAA;\nCN,10,3,39064,1,10,0,0,10;\nAA;\nCN,10,3,39455,1,10,0,0,10;\nAA;\nCN,10,3,39850,1,10,0,0,10;\nAA;\nCN,10,3,40248,1,10,0,0,10;\nAA;\nCN,10,3,40650,1,10,0,0,10;\nAA;\nCN,10,3,41056,1,10,0,0,10;\nAA;\nCN,10,3,41467,1,10,0,0,10;\nAA;\nCN,10,3,41882,1,10,0,0,10;\nAA;\nCN,10,3,42301,1,10,0,0,10;\nAA;\nCN,10,3,42724,1,10,0,0,10;\nAA;\nCN,10,3,43151,1,10,0,0,10;\nAA;\nCN,10,3,43583,1,10,0,0,10;\nAA;\nCN,10,3,44019,1,10,0,0,10;\nAA;\nCN,10,3,44459,1,10,0,0,10;\nAA;\nCN,10,3,44904,1,10,0,0,10;\nAA;\nCN,10,3,45353,1,10,0,0,10;\nAA;\nCN,10,3,45807,1,10,0,0,10;\nAA;\nCN,10,3,46265,1,10,0,0,10;\nAA;\nCN,10,3,46728,1,10,0,0,10;\nAA;\nCN,10,3,47195,1,10,0,0,10;\nAA;\nCN,10,3,47667,1,10,0,0,10;\nAA;\nCN,10,3,48144,1,10,0,0,10;\nAA;\nCN,10,3,48625,1,10,0,0,10;\nAA;\nCN,10,3,49111,1,10,0,0,10;\nAA;\nCN,10,3,49602,1,10,0,0,10;\nAA;\nCN,10,3,50098,1,10,0,0,10;\nAA;\nCN,10,3,50599,1,10,0,0,10;\nAA;\nCN,10,3,51105,1,10,0,0,10;\nAA;\nCN,10,3,51616,1,10,0,0,10;\nAA;\nCN,10,3,52132,1,10,0,0,10;\nAA;\nCN,10,3,52653,1,10,0,0,10;\nAA;\nCN,10,3,53180,1,10,0,0,10;\nAA;\nCN,10,3,53712,1,10,0,0,10;\nAA;\nCN,10,3,54249,1,10,0,0,10;\nAA;\nCN,10,3,54791,1,10,0,0,10;\nAA;\nCN,10,3,55339,1,10,0,0,10;\nAA;\nCN,10,3,55892,1,10,0,0,10;\nAA;\nCN,10,3,56451,1,10,0,0,10;\nAA;\nCN,10,3,57016,1,10,0,0,10;\nAA;\nCN,10,3,57586,1,10,0,0,10;\nAA;\nCN,10,3,58162,1,10,0,0,10;\nAA;\nCN,10,3,58744,1,10,0,0,10;\nAA;\nCN,10,3,59331,1,10,0,0,10;\nAA;\nCN,10,3,59924,1,10,0,0,10;\nAA;\nCN,10,3,60523,1,10,0,0,10;\nAA;\nCN,10,3,61128,1,10,0,0,10;\nAA;\nCN,10,3,61739,1,10,0,0,10;\nAA;\nCN,10,3,62356,1,10,0,0,10;\nAA;\nCN,10,3,62980,1,10,0,0,10;\nAA;\nCN,10,3,63610,1,10,0,0,10;\nAA;\nCN,10,3,64246,1,10,0,0,10;\nAA;\nCN,10,3,64888,1,10,0,0,10;\nAA;\nCN,10,3,65537,1,10,0,0,10;\nAA;\nCN,10,3,66192,1,10,0,0,10;\nAA;\nCN,10,3,66854,1,10,0,0,10;\nAA;\nCN,10,3,67523,1,10,0,0,10;\nAA;\nCN,10,3,68198,1,10,0,0,10;\nAA;\nCN,10,3,68880,1,10,0,0,10;\nAA;\nCN,10,3,69569,1,10,0,0,10;\nAA;\nCN,10,3,70265,1,10,0,0,10;\nAA;\nCN,10,3,70968,1,10,0,0,10;\nAA;\nCN,10,3,71678,1,10,0,0,10;\nAA;\nCN,10,3,72395,1,10,0,0,10;\nAA;\nCN,10,3,73119,1,10,0,0,10;\nAA;\nCN,10,3,73850,1,10,0,0,10;\nAA;\nCN,10,3,74588,1,10,0,0,10;\nAA;\nCN,10,3,75334,1,10,0,0,10;\nAA;\nCN,10,3,76087,1,10,0,0,10;\nAA;\nCN,10,3,76848,1,10,0,0,10;\nAA;\nCN,10,3,77616,1,10,0,0,10;\nAA;\nCN,10,3,78392,1,10,0,0,10;\nAA;\nCN,10,3,79176,1,10,0,0,10;\nAA;\nCN,10,3,79968,1,10,0,0,10;\nAA;\nCN,10,3,80000,1,10,0,0,10;\nAA;\nAR;" ("Commandlist")) -> ("outputstring"=w6:string)  [unwired: 10 in]
      n27 = call-dynamic "set wait.vi"("error in (no error)"=w42, "wait"=i32[] [1200], "TestInterface in"=w43) -> ("error out"=w45:errorcluster, "TestInterface out"=w44:refnum<class "HF-Felder.lvclass">)  [unwired: 7 in]
      n28 = call-dynamic "set Commandlist.vi"("error in (no error)"=w45, "Commandlist"=w6, "TestInterface (Eingang)"=w44) -> ("error out"=w77:errorcluster, "TestInterface (Ausgang)"=w79:refnum<class "HF-Felder.lvclass">)  [unwired: 7 in]
      n29 = Build Array(w55, w64, w79) -> (w78:refnum<class "HF-Felder.lvclass">[])
      n30 = call-dynamic "add Tests.vi"("error in (no error)"=w77, "Tests"=w78, "DeviceInterface (Eingang)"=w75) -> ("error out"=w76:errorcluster, "DeviceInterface (Ausgang)"=w74:refnum<class "EMTestCWS500N.lvclass">)  [unwired: 7 in]
    }
    frame Error {
    }
  }
  "error out" <- w4
  "EMTestCWS500N Ausgang" <- w1
